vi "WVDIAL_2_OphirPM_v2.2_temp_tune.vi"() -> ()   [LabVIEW 2012]
uses:
  <vilib>/DAQmx/write.llb/DAQmx Write (Digital 1D Bool NChan 1Samp 1Line).vi
  <vilib>/DAQmx/miscellaneous.llb/DAQmx Fill In Error Info.vi
  under_development/AMCS_Data.vi
  <vilib>/Analysis/baseanly.llb/Mean (DBL).vi
  H2O_DIAL/LabVIEW-2012/Scalar_Data.vi
  H2O_DIAL/LabVIEW-2012/Bristol WM V2_31b/CLDevIFace.dll
  <vilib>/Analysis/NI_AALBase.lvlib
panel:
  out "AMCS_Profile":i32=256
  out "FileHour":i32=14
  out "L_Count":i32=93
  out "sigma_off_total":dbl[](array[numeric])=[5.314422064744898e-25, 5.279415210171283e-25, 5.244590126473598e-25, 5.20994645782043e-25, 5.175483839803292e-25, 5.1412018994858e-25, 5.1071002554464015e-25, 5.073178517853386e-25, 5.03943628848111e-25, 5.00587316081542e-25, 4.972488720065558e-25, 4.939282543255047e-25, 4.906254199251138e-25, 4.873403248837318e-25, 4.840729244783645e-25, 4.808231731862337e-25, 4.775910246962909e-25, 4.743764319119939e-25, 4.711793469569763e-25, 4.67999721182007e-25, 4.648375051724865e-25, 4.616926487509067e-25, 4.585651009873473e-25, 4.5545481020267065e-25, 4.52361723976039e-25, 4.49285789150236e-25, 4.4622695183981935e-25, 4.4318515743427665e-25, 4.40160350608453e-25, 4.371524753261039e-25, 4.3416147484733715e-25, 4.311872917347073e-25, 4.282298678608985e-25, 4.252891444145085e-25, 4.223650619059866e-25, 4.194575601773045e-25, 4.1656657840359355e-25, 4.136920551058964e-25, 4.1083392815469774e-25, 4.0799213477702186e-25, 4.05166611564624e-25, 4.0235729448119603e-25, 3.9956411886755236e-25, 3.967870194537133e-25, 3.9402593036058175e-25, 3.9128078511145925e-25, 3.885515166392363e-25, 3.858380572923638e-25, 3.8314033884573097e-25, 3.804582925057902e-25, 3.777918489222167e-25, 3.7514093819211588e-25, 3.7250548987302515e-25, 3.698854329879953e-25, 3.6728069603748863e-25, 3.646912070062639e-25, 3.62116893374067e-25, 3.595576821249159e-25, 3.5701349975624987e-25, 3.54484272290085e-25, 3.519699252824005e-25, 3.4947038383229287e-25, 3.469855725968371e-25, 3.445154157974239e-25, 3.420598372340985e-25, 3.3961876029492998e-25, 3.3719210796961754e-25, 3.347798028606905e-25, 3.323817671960307e-25, 3.2999792284274424e-25, 3.276281913173581e-25, 3.2527249380236306e-25, 3.2293075115830613e-25, 3.2060288393816585e-25, 3.1828881240106345e-25, 3.1598845652910105e-25, 3.1370173603985285e-25, 3.1142857040280253e-25, 3.091688788564397e-25, 3.069225804235743e-25, 3.0468959392679594e-25, 3.0246983800716816e-25, 3.002632311398086e-25, 2.980696916543016e-25, 2.958891377497247e-25, 2.9372148751466003e-25, 2.9156665894504283e-25, 2.89424569964799e-25, 2.8729513844353943e-25, 2.8517828221847843e-25, 2.8307391911095345e-25, 2.8098196695181605e-25, 2.7890234359787145e-25, 2.768349669545398e-25, 2.7477975499672548e-25, 2.727366257913024e-25, 2.7070549751927695e-25, 2.6868628849298454e-25, 2.6667891718580697e-25, 2.6468330224752645e-25, 2.6269936253020695e-25, 2.6072701711097747e-25, 2.587661853105292e-25, 2.5681678672237707e-25, 2.5487874122831935e-25, 2.529519690252841e-25, 2.5103639064422395e-25, 2.491319269774056e-25, 2.4723849929592074e-25, 2.453560292702316e-25, 2.434844389973349e-25, 2.416236510156665e-25, 2.3977358833193057e-25, 2.379341744342703e-25, 2.3610533331668965e-25, 2.3428698949963e-25, 2.3247906804276327e-25, 2.3068149456696086e-25, 2.288941952726386e-25, 2.2711709695222057e-25, 2.2535012700704786e-25, 2.235932134638202e-25, 2.21846284987704e-25, 2.201092708924474e-25, 2.183821011536941e-25, 2.1666470642157234e-25, 2.1495701802684266e-25, 2.1325896798994203e-25, 2.1157048902866705e-25, 2.098915145620556e-25, 2.082219787182239e-25, 2.0656181633016752e-25, 2.0491096294692994e-25, 2.0326935482406903e-25, 2.016369289258156e-25, 2.000136229269397e-25, 1.9839937520011981e-25, 1.9679412481191304e-25, 1.9519781152122327e-25, 1.9361037576226607e-25, 1.9203175863925343e-25, 1.9046190191099535e-25, 1.889007479817365e-25, 1.8734823987870487e-25, 1.8580432124512337e-25, 1.8426893631518894e-25, 1.8274202989506262e-25, 1.8122354735223218e-25, 1.7971343458200367e-25, 1.7821163799049579e-25, 1.767181044716152e-25, 1.752327813814955e-25, 1.737556165177881e-25, 1.7228655808367516e-25, 1.7082555467277782e-25, 1.693725552343894e-25, 1.6792750905240115e-25, 1.6649036571579248e-25, 1.650610750886898e-25, 1.6363958728621502e-25, 1.622258526492432e-25, 1.6081982171721664e-25, 1.594214451997735e-25, 1.580306739598529e-25, 1.5664745897902764e-25, 1.5527175135035033e-25, 1.5390350223941979e-25, 1.5254266288135843e-25, 1.5118918456024445e-25, 1.4984301858342265e-25, 1.4850411628570882e-25, 1.4717242900420903e-25, 1.4584790807687737e-25, 1.4453050483797776e-25, 1.4322017062029086e-25, 1.4191685674596558e-25, 1.4062051453739477e-25, 1.3933109532543182e-25, 1.3804855046380026e-25, 1.367728313352582e-25, 1.35503889384992e-25, 1.3424167612815224e-25, 1.3298614318833922e-25, 1.3173724233032037e-25, 1.3049492548807338e-25, 1.2925914480776576e-25, 1.2802985269669848e-25, 1.268070018646981e-25, 1.2559054538186517e-25, 1.2438043673528122e-25, 1.231766298852889e-25, 1.2197907933722819e-25, 1.207877402055392e-25, 1.1960256828031697e-25, 1.1842352011821407e-25, 1.172505531033491e-25, 1.160836255409088e-25, 1.149226967367832e-25, 1.1376772708317697e-25, 1.1261867814713535e-25, 1.1147551275979209e-25, 1.1033819510978471e-25, 1.0920669083258334e-25, 1.0808096709575008e-25, 1.069609927077414e-25, 1.0584673818555839e-25, 1.0473817586142326e-25, 1.0363527996489042e-25, 1.0253802670476093e-25, 1.0144639436397076e-25, 1.0036036335541817e-25, 9.927991632011449e-26, 9.820503819270136e-26, 9.713571625261393e-26, 9.607194020823438e-26, 9.501370223040411e-26, 9.396099700993619e-26, 9.291382180414976e-26, 9.187217645653203e-26, 9.083606343720884e-26, 8.980548784653646e-26, 8.878045744250468e-26, 8.776098262714437e-26, 8.674707644122939e-26, 8.573875455102998e-26, 8.473603522131269e-26, 8.373893928088327e-26, 8.274749007134821e-26, 8.17617134051572e-26, 8.078163749082583e-26, 7.980729286044041e-26, 7.883871229773624e-26, 7.78759307512813e-26, 7.691898521304032e-26, 7.596791464219395e-26, 7.502275983080843e-26, 7.408356329263953e-26, 7.315036913619158e-26, 7.222322292848408e-26, 7.130217155120976e-26, 7.038726307749827e-26, 6.947854659579743e-26, 6.857607208469795e-26, 6.767989024717408e-26, 6.679005234677889e-26, 6.59066100689568e-26, 6.502961534631894e-26, 6.415912020823876e-26, 6.329517661488074e-26, 6.243783631897422e-26, 6.158715068187244e-26, 6.074317054761003e-26, 5.99059460805025e-26, 5.907552662478026e-26, 5.825196055341633e-26, 5.743529514672476e-26, 5.662557645089932e-26, 5.582284915282987e-26, 5.502715646791743e-26, 5.423854001499785e-26, 5.345703972449223e-26, 5.268269372490484e-26, 5.191553826272697e-26, 5.1155607608625183e-26, 5.040293398726036e-26, 4.965754750357786e-26, 4.891947608760883e-26, 4.818874542569047e-26, 4.7465378935362823e-26, 4.674939770825742e-26, 4.604082049111456e-26, 4.533966365256215e-26, 4.464594117661327e-26, 4.395966464565719e-26, 4.328084324397715e-26, 4.260948375846483e-26, 4.1945590589570554e-26]
  out "sigma_on_total":dbl[](array[numeric])=[1.3869479575219666e-23, 1.3807437011066577e-23, 1.37449636602892e-23, 1.3682071082128486e-23, 1.3618770829571316e-23, 1.3555074444096617e-23, 1.3490993450978266e-23, 1.3426539354204636e-23, 1.3361723632425733e-23, 1.3296557734520282e-23, 1.3231053075022487e-23, 1.3165221030343146e-23, 1.3099072933460705e-23, 1.303262007172832e-23, 1.2965873680839169e-23, 1.2898844942369238e-23, 1.2831544980028457e-23, 1.2763984855328133e-23, 1.269617556404732e-23, 1.2628128033261598e-23, 1.2559853118242374e-23, 1.2491361598101514e-23, 1.2422664174044883e-23, 1.23537714654586e-23, 1.2284694007241841e-23, 1.221544224679423e-23, 1.2146026542230557e-23, 1.2076457158241087e-23, 1.2006744265409983e-23, 1.1936897936295945e-23, 1.1866928144067788e-23, 1.1796844760131547e-23, 1.1726657551867315e-23, 1.1656376181342888e-23, 1.1586010202384198e-23, 1.1515569060143322e-23, 1.1445062087730294e-23, 1.137449850683545e-23, 1.1303887424350273e-23, 1.1233237832313931e-23, 1.1162558605600282e-23, 1.1091858502038009e-23, 1.1021146159869723e-23, 1.0950430098256995e-23, 1.0879718715139568e-23, 1.0809020287073718e-23, 1.0738342968727736e-23, 1.0667694791434451e-23, 1.0597083663475774e-23, 1.0526517369210098e-23, 1.0456003568894101e-23, 1.0385549797974356e-23, 1.0315163467461895e-23, 1.024485186317274e-23, 1.0174622145845567e-23, 1.0104481351323143e-23, 1.003443639040392e-23, 9.964494049153228e-24, 9.89466098849997e-24, 9.824943745255963e-24, 9.755348732024939e-24, 9.685882237371367e-24, 9.616550426617036e-24, 9.547359341927676e-24, 9.47831490321052e-24, 9.40942290830694e-24, 9.340689033982913e-24, 9.272118836219597e-24, 9.203717751107802e-24, 9.135491095777061e-24, 9.067444068641131e-24, 8.999581750772038e-24, 8.931909106582237e-24, 8.864430984196331e-24, 8.797152117625856e-24, 8.730077126495636e-24, 8.663210517401465e-24, 8.596556685453482e-24, 8.530119914634811e-24, 8.46390437922709e-24, 8.397914144742156e-24, 8.332153169383828e-24, 8.266625304687613e-24, 8.201334296859706e-24, 8.136283788452192e-24, 8.071477318738257e-24, 8.006918325585158e-24, 7.942610146035729e-24, 7.878556018198735e-24, 7.81475908249396e-24, 7.751222382124728e-24, 7.687948864992263e-24, 7.624941385280568e-24, 7.562202703660279e-24, 7.499735489821076e-24, 7.43754232269632e-24, 7.375625692531723e-24, 7.31398800203366e-24, 7.25263156693754e-24, 7.191558618654768e-24, 7.130771304396952e-24, 7.070271689077592e-24, 7.010061756330106e-24, 6.950143409961645e-24, 6.890518475536768e-24, 6.831188701248949e-24, 6.772155758945719e-24, 6.713421246257091e-24, 6.654986687320795e-24, 6.596853534201044e-24, 6.539023168026952e-24, 6.481496900395139e-24, 6.424275974626182e-24, 6.3673615670133464e-24, 6.310754787803715e-24, 6.254456682823536e-24, 6.198468234566776e-24, 6.142790363279649e-24, 6.087423928166582e-24, 6.032369728708771e-24, 5.977628505719948e-24, 5.923200942640215e-24, 5.869087666691756e-24, 5.815289249902529e-24, 5.761806210124825e-24, 5.708639012516363e-24, 5.655788070409e-24, 5.603253746407087e-24, 5.551036353473567e-24, 5.4991361562284445e-24, 5.447553371437421e-24, 5.396288169850396e-24, 5.345340676553168e-24, 5.2947109721049526e-24, 5.244399093980751e-24, 5.1944050370119895e-24, 5.1447287546918326e-24, 5.09537016002838e-24, 5.0463291264942426e-24, 4.9976054888585635e-24, 4.949199044317764e-24, 4.901109553397718e-24, 4.853336740542285e-24, 4.805880295200359e-24, 4.758739872789894e-24, 4.711915095350015e-24, 4.6654055524798795e-24, 4.619210802353354e-24, 4.5733303718584396e-24, 4.527763758259087e-24, 4.482510429403448e-24, 4.437569824594334e-24, 4.392941355621808e-24, 4.3486244071369034e-24, 4.304618337478862e-24, 4.260922479571828e-24, 4.217536141448475e-24, 4.174458607031095e-24, 4.13168913672264e-24, 4.0892269680759445e-24, 4.0470713165327956e-24, 4.0052213761463945e-24, 3.96367631979338e-24, 3.9224353003739355e-24, 3.8814974509190375e-24, 3.840861885432312e-24, 3.800527699468413e-24, 3.760493970621977e-24, 3.72075975901009e-24, 3.681324108052961e-24, 3.642186044776093e-24, 3.603344580489083e-24, 3.564798711222146e-24, 3.526547418229872e-24, 3.4885896684839234e-24, 3.4509244152268236e-24, 3.413550598298677e-24, 3.376467144672314e-24, 3.339672968905001e-24, 3.3031669737165538e-24, 3.2669480501429536e-24, 3.231015078099695e-24, 3.1953669267941692e-24, 3.1600024551943975e-24, 3.1249205122895757e-24, 3.0901199376068864e-24, 3.055599561330377e-24, 3.0213582050544584e-24, 2.987394681822326e-24, 2.953707796666617e-24, 2.92029634676618e-24, 2.8871591220256764e-24, 2.854294905098644e-24, 2.821702472007482e-24, 2.7893805922154235e-24, 2.7573280291639967e-24, 2.725543540222118e-24, 2.694025877377622e-24, 2.662773787176486e-24, 2.6317860112783244e-24, 2.60106128650067e-24, 2.5705983450847046e-24, 2.5403959152174938e-24, 2.5104527209047027e-24, 2.4807674825825997e-24, 2.4513389169868365e-24, 2.4221657375927964e-24, 2.3932466549360318e-24, 2.3645803764788273e-24, 2.3361656072702794e-24, 2.308001049756091e-24, 2.2800854041775233e-24, 2.2524173687645203e-24, 2.2249956398311676e-24, 2.197818912100556e-24, 2.170885878654516e-24, 2.1441952314281124e-24, 2.1177456610619372e-24, 2.091535857292432e-24, 2.065564508979104e-24, 2.0398303043057066e-24, 2.014331931015518e-24, 1.9890680763476753e-24, 1.9640374273914704e-24, 1.9392386711399865e-24, 1.9146704945060966e-24, 1.890331584774096e-24, 1.8662206293279557e-24, 1.8423363160920896e-24, 1.8186773334553743e-24, 1.795242370503451e-24, 1.7720301170920184e-24, 1.749039263883513e-24, 1.7262685025646166e-24, 1.703716525946266e-24, 1.6813820279212657e-24, 1.6592637036703435e-24, 1.6373602498566653e-24, 1.6156703644751474e-24, 1.5941927471134708e-24, 1.572926098969147e-24, 1.5518691229974072e-24, 1.5310205238931107e-24, 1.510379008202476e-24, 1.48994328452232e-24, 1.4697120633218853e-24, 1.44968405723214e-24, 1.4298579810194845e-24, 1.410232551681262e-24, 1.3908064884217362e-24, 1.371578512888116e-24, 1.3525473490547908e-24, 1.333711723340262e-24, 1.315070364690135e-24, 1.2966220046291443e-24, 1.2783653772848224e-24, 1.2602992193856838e-24, 1.2424222704417105e-24, 1.2247332727096541e-24, 1.207230971188227e-24, 1.1899141137880397e-24, 1.1727814512227674e-24, 1.1558317371980456e-24, 1.1390637283275014e-24, 1.1224761842431351e-24, 1.1060678675840506e-24, 1.0898375441228311e-24, 1.0737839826609285e-24, 1.057905955131391e-24, 1.0422022366512468e-24, 1.0266716055496742e-24, 1.0113128433115541e-24, 9.96124734733142e-25, 9.811060678425485e-25, 9.662556339483166e-25, 9.515722277242587e-25, 9.370546471719464e-25]
  out "background start":u32=254
  in  "Tab Control 2":enum32{"WV ND Narrow", "WV ND Wide"}(tab)
  out "Water Vapor Number Density":dbl[][](graph)=[[2.6979991604572735, 2.9593143915657074, 2.797449584571317, 2.404658952819358, 2.3195212072555154, 2.5116972565306184, 2.4617308913751637, 2.4391959235044225, 2.6692800938976244, 2.741253898038124, 2.644730576020495, 2.3610708500867044, 2.1476349969634225, 2.2002457128655424, 2.4968510217618705, 2.554578876255192, 2.0454846988586315, 1.8023042055354455, 1.9720735301407404, 1.8926202748500127, 1.7837401064253728, 2.0676382839883733, 2.08031025810689, 1.773643007504944, 1.6546102834122778, 1.6279557460647043, 1.6011324659921025, 1.0021875680291408, 0.41374082119247085, 0.4527192082231668, 2.3516701899198997, 4.374135424821069, 0.39214939184879105, -5.085477705081822, -0.6454633347922013, 8.345959457204707, 1.182839582693342, -1.7003003047291725, 6.536266318699054, -2.327645608957367, 2.797319081322348, 0.10721086091200081, 0.8678650894368296, -0.292961171425824, -1.2405862868143065, 0.08002385618879078, 1.1423277801066902, 0.8810874015440164, 1.166620200538605, 1.1437670100476367, 3.3905729378505236, 5.02328449196602, 2.4176112321239813, 1.7373231866673655, 0.21866881048224668, -0.6606779691744664, 0.8866008233295397, 5.183030048638962, 7.624360936578197, -2.561027107157697, -4.6351658542352805, -4.1844318407939305, -2.990804811815481, -0.08651792227088426, 2.1460065959464, 5.64031573417192, 7.404702135500966, 1.3666150911852348, -7.13957308573761, 0.3596983598284657, -3.2319741125605272, -5.382731401201804, -3.658947755685539, -6.466561447894286, -2.5894001538271456, -3.5936030711328533, -9.45888310637412, 5.337453776109291, 2.523301465289049, -0.4444154792139517, 3.9416736698791515, -0.31355796660419666, -1.8373168582667905, 0.9955190223681669, -1.089077347483283, -6.281856233414937, 6.257260372926666, -13.655858715766612, 5.830204522057969, 9.609389261892614, -3.924288936198821, 4.924456138151559, 4.670517947496226, 7.722670563052783, 12.254047544716892, 9.745839454508765, -3.8105997194228154, 0.4890661768678136, 11.894606542817344, -16.259140432303216, 12.884851240924808, -9.074814833037872, -0.07410598267861004, 13.032695980210102, -15.347711948234926, -2.2813575808650772, -0.37180440848685486, 19.946704578086855, -16.686062841021247, -9.894667631120459, -20.995606668812822, -2.2526592621705586, -16.3908377368364, -21.31038895828113, 32.72210513307602, -9.717538636026543, -9.890235552804324, -26.917838345809066, -11.15341741047493, 16.822178540332708, 11.164934912668619, 8.976059522967718, 16.44419788472998, 5.521276634043085, -27.348050690597656, 3.2607914106748015, 10.64540411389454, 26.35964743727274, 8.217737459322414, -2.1446882284347537, -1.6240017477306874, 0.8694361012620837, 0.2753212901219622, -2.017177128570476, -1.7367818265406356, 2.738866245516143, -2.2576465932228675, -18.144499153577325, -3.4713944166922777, 0.025358387211094534, 3.8925246272702494, 2.6620676732061166, -5.242800367205337, -4.258745982226573, -0.746059052925772, -0.05154706973106406, 2.990291161294011, 8.0729458717512, 8.116266129237458, 6.226968559806926, -17.485848033155328, -7.175474933960434, 9.897116918290264, -5.562391740806701, -28.26312520479269, -37.18466121475089, 3.0379212507936595, -49.25326375258036, -49.55319390746631, -75.79505294806995, -31.800298571915437, -21.323573928947045, 6.170114127015452, -32.59512054829957, 41.14643545755569, 72.32002090526684, -19.19621968895502, 76.64601181450533, 40.58764334357079, 43.20212176036005, 30.51415344385976, -18.900153250831522, -12.69555435106068, 40.90487604463205, -43.90464231635574, -71.87217734267412, -85.25284930724254, -98.86218389373931, -37.211623515974594, -4.660221249767364, -8.30223960482317, -78.11880710674619, -52.936142176356334, 10.739065034224021, 27.17659341050922, 43.27549838133942, 78.6390303110269, 31.63798764245529, 22.840921363665966, -15.424992732340193, -67.11504703685894, 95.28139075009446, 47.665759432899335, 39.75623750944128, 12.07897488147926, -13.595402683839163, -16.244355600957185, 39.56289276585016, -58.46898177728697, -5.705909600699701, 36.35847497013099, -103.67852139769494, -65.209907256163, -117.84105778782569, -37.196968834476365, -4.511454495944519, 38.957598425261125, -28.163785822065798, 55.90715401535311, 20.281060958402115, 100.0959062964011, 29.293400539831783, 55.15876114229656, -65.2961513762635, -4.429021621104553, -22.382554280854816, 15.842494942030372, -29.55499174522829, 7.668766094225895, 50.010508877808284, -88.02683061785386, 30.08347486970615, 106.39829367365633, 145.2321906759042, -1.858002730325935, -18.46040484465744, 1.3292343668491104, 29.845298073762176, 20.54006800357979, 6.775417401267568, 108.55704162770199, 21.35361701301774, -22.183740735151503, 26.424235225087745, -0.2082268013256196, 11.16104876593104, 74.9397615826961, 0.2512828787561202, -18.73257114374409, -9.174859609068479, -0.6049319170897494, 41.81659884060494, -105.33239517840579, -50.40203588046909, 294.29886187228936, 68.70660941139782, -104.26441281434118, -17.894724880282443, -14.734992121972157, -79.59667884368375, -149.05753799401518, 30.40850937412097, -4.110243462106567, -30.737568940274127, -355.33349697162674, -84.80653337159367, 60.380833898611876, -72.78540457827825, -55.41791512520111, -117.56784011631594, 73.39110087767413, 236.13722109125632, -50.17444896136822, 72.78920342275046, -77.32879365741358, -50.85238879922648, -149.21416360461436, 57.54491199600477, 205.8524361343854, 232.8390700997829, -110.53199462104917, -378.03756929059244, -27.712093052120554, -149.1541222983105, 54.68721852689611, -11.376835333855148, 0.0, 0.0, 0.0, 0.0]]
  out "Water Vapor Number Density 2":dbl[][](graph)=[[nan, nan, nan, nan, nan, nan, nan, nan, nan, nan, nan, nan, nan, nan, nan, nan, nan, nan, nan, nan, nan, nan, nan, nan, nan, nan, nan, nan, nan, nan, nan, nan, nan, nan, nan, nan, nan, nan, nan, nan, nan, nan, nan, nan, nan, nan, nan, nan, nan, nan, nan, nan, nan, nan, nan, nan, nan, nan, nan, nan, nan, nan, nan, nan, nan, nan, nan, nan, nan, nan, nan, nan, nan, nan, nan, nan, nan, nan, nan, nan, nan, nan, nan, nan, nan, nan, nan, nan, nan, nan, nan, nan, nan, nan, nan, nan, nan, nan, nan, nan, nan, nan, nan, nan, nan, nan, nan, nan, nan, nan, nan, nan, nan, nan, nan, nan, nan, nan, nan, nan, nan, nan, nan, nan, nan, nan, nan, nan, nan, nan, nan, nan, nan, nan, nan, nan, nan, nan, nan, nan, nan, nan, nan, nan, nan, nan, nan, nan, nan, nan, nan, nan, nan, nan, nan, nan, nan, nan, nan, nan, nan, nan, nan, nan, nan, nan, nan, nan, nan, nan, nan, nan, nan, nan, nan, nan, nan, nan, nan, nan, nan, nan, nan, nan, nan, nan, nan, nan, nan, nan, nan, nan, nan, nan, nan, nan, nan, nan, nan, nan, nan, nan, nan, nan, nan, nan, nan, nan, nan, nan, nan, nan, nan, nan, nan, nan, nan, nan, nan, nan, nan, nan, nan, nan, nan, nan, nan, nan, nan, nan, nan, nan, nan, nan, nan, nan, nan, nan, nan, nan, nan, nan, nan, nan, nan, nan, nan, nan, nan, nan, nan, nan, nan, nan, nan, nan, nan, nan, nan, nan, nan, nan, nan, nan, nan, nan, nan, nan, nan, nan, nan, nan, nan, nan, nan, nan, 0.0, 0.0, 0.0, 0.0]] caption="Water Vapor Number Density"
  out "RingBuffer offline near":dbl[][](array[numeric])
  out "RingBuffer aerosol near":dbl[][](array[numeric])
  in  "LOWER DISPLAY TAB":T1(tab)=enum."Raw Counts Narrow"
  out "NRB":dbl[][](graph)=[[0.00046653927091916777, 0.0026614448003019955, 0.00799000665119036, 0.017338442995885873, 0.030659739318508464, 0.048690127127963834, 0.07257190803169539, 0.1022875233425713, 0.13895426462578678, 0.18353308368702612, 0.2374733807532343, 0.29827916455644055, 0.36303037111961745, 0.4387277399880996, 0.5296240484959289, 0.6448056167411246, 0.7968692742688123, 0.986211936517738, 1.2272580015909782, 1.5045937819461137, 1.6804030717427192, 1.6930670107515053, 1.7186662137889164, 1.8220745936144405, 1.921986223781103, 2.0763561968674273, 2.2958981573467914, 2.3486417326554654, 2.047301484620606, 1.411776366563831, 0.7124512356303606, 0.3105075790623782, 0.2141663700100353, 0.2121969246397393, 0.19959202927447903, 0.1761001939839144, 0.16578999175180362, 0.17348619277005686, 0.17737239738890392, 0.19260470674885563, 0.18387703555551488, 0.1683847338008346, 0.18113483921557574, 0.19140229669855557, 0.20519979528052695, 0.23908830659210373, 0.24929346127216373, 0.21410890747194383, 0.19758618909133507, 0.19339446633371923, 0.1918349029632283, 0.1666024208595111, 0.17274180772746983, 0.18857177921404147, 0.16091218794964157, 0.15551975294417666, 0.19172069794668137, 0.21550100504467, 0.1939605427805015, 0.15555508504784912, 0.15837969068596502, 0.17392434388819766, 0.17375269565396587, 0.18099628966643178, 0.1552686332629994, 0.1871983829024575, 0.19326554001157917, 0.1759961805666762, 0.20702641454615772, 0.17230592991361512, 0.15624762843920986, 0.1362276160575669, 0.11219171781224463, 0.16126344429341657, 0.17622056993508411, 0.13652363159974298, 0.13828342852020437, 0.13106340939532152, 0.13053713937048633, 0.1098155705898619, 0.12618801482529873, 0.16498428580884197, 0.16768457837801556, 0.1613926144792111, 0.1467353339521328, 0.14687923449528653, 0.09921420381956712, 0.028623899549958025, 0.09638828573179213, 0.13898533152779396, 0.0993106431198225, 0.1341337314641019, 0.08578445870698116, 0.14988499019441937, 0.24740804086795487, 0.23532835084484116, 0.1365893927881256, 0.09149807112681532, 0.16145936216816204, 0.17178252103390232, 0.15986434455570978, 0.10909509408905861, 0.11830283727003509, 0.09754229119527288, 0.0629700043568801, 0.16201238738941418, 0.1861436261348872, 0.21566036035440786, 0.19200480679779117, 0.1462942034668786, 0.19646330323797864, 0.17424490794472436, 0.24358767939255435, 0.15560140404548056, -0.03262194064558316, -0.05030318579422492, 0.063722224941549, -0.0016563122467756772, -0.02246353446437762, 0.10337828990755542, 0.1116973847636031, 0.1441309624918215, 0.12962967679387316, 0.13565725674439336, 0.04155142740366882, 0.3597156443785714, 0.9053359221232993, 1.3274351658049444, 1.5516506598520667, 1.6890247548740251, 1.456939178163056, 0.8251997771899959, 0.5264651467937713, 0.5474151217059147, 1.153592838836607, 2.7245958688554976, 5.9590100032700875, 10.358807868304037, 13.752597951922784, 13.321173266620074, 9.929368166634307, 8.319699656050076, 10.215466411241565, 11.264037378065957, 8.239090023036898, 3.8676449804333157, 1.8091720120289554, 1.5417339483555401, 1.184874433985245, 1.1964269980813527, 1.8071508438115211, 2.8350889457012673, 3.31983490827713, 2.551437870592605, 1.1740390978029294, 0.4566254679466681, 0.14705412703589116, 0.1748216055487878, 0.19336548065559225, -0.10070999224246821, -0.00916904547514361, 0.05489969276362185, -0.0613790147296684, -0.008461508611298307, 0.10489231744081019, 0.2253241019004552, 0.2744321054481327, 0.1556808399563599, 0.14133368334941515, 0.10060220872991148, 0.09835652831180781, 0.31658200601100306, 0.47195886105167817, 0.4276641830684275, 0.15394419938215426, -0.03701654742796507, 0.0630851327862899, -0.039102373767677445, 0.10652094665295668, 0.10264304191186455, 0.18839860179433146, 0.2377987829790185, -0.1337107048088187, 0.009220418178048348, 0.041462246018112034, -0.10564267279908282, 0.12514963530437614, 0.013774666881661655, -0.30544644422181294, -0.08551608415499386, 0.10272375530400045, 0.19251893526497038, 0.319889127727876, -0.06632874219283735, -0.3987896018285478, -0.017346889667260754, 0.41454046411268386, 0.4287323252398325, 0.27654890615479055, 0.0069807213602538455, 0.052106026597721615, 0.07897094487093263, -0.0694008008611362, -0.17674330597107643, -0.14394925906419756, 0.13443704094357667, 0.31851437756105405, -0.03985065387486617, -0.3248039530724683, 0.008559054170191926, 0.08529365932724306, 0.09225944268644928, -0.016936024365819886, 0.2839683030158373, 0.44400723102129164, 0.1797559582192265, 0.24776078000505974, -0.14047093671496036, -0.4898589719637731, -0.03321834143453104, 0.2225764985272629, 0.12141788420013612, 0.23732622403377998, 0.3091639446236378, 0.37037323028296343, 0.13182866468330257, -0.08073210235332377, -0.0895812330679099, -0.08729083537973405, 0.17172702391260303, 0.06151272265106227, 0.11785957903150333, 0.27183497399482814, 0.5377361440387042, 0.2894881510858271, 0.009719956422017425, 0.23179347279449192, -0.18959136484778202, -0.27164793180882657, 0.11035050374540555, 0.03627218441554687, -0.5729506651960073, -0.7197745629796234, -0.5020978864046269, -0.26197225331804413, -0.2842416644426923, -0.12303750456090687, -0.03860209607355206, -0.20873459471373904, 0.106286853878823, 0.056601357578755326, -0.20634031751796159, 0.3367860809816278, 0.360913317766556, 0.052058689588379094, -0.05139020644874281, -0.19781130293363244, -0.14856534214258266, 0.005144708507677107, 0.20622067097216687, 0.1691582294324484, 0.33565453726380606, 0.30032763979924, -0.4228041465415953, -0.586748613218039, 0.10509902204196496, -0.15353229797165785, -0.7209430470045907, -0.1827390073296543, 0.11113626218212269, -0.24868566608054246, 0.13450151047086945, 0.4665084611774521, 0.30834835440009084, -0.14067735872021378, -0.35630589536410423, 0.046416854918681326, 0.0, 0.0, 0.0]] caption="Water Vapor Number Density"
  out "NRB 2":dbl[][](graph) caption="Water Vapor Number Density"
  out "raw counts":dbl[][](graph)=[[342.03999999999996, 498.03999999999996, 667.04, 800.04, 1022.04, 1083.04, 1284.04, 1434.04, 1514.04, 1579.04, 1641.04, 1669.04, 1825.04, 1971.04, 1925.04, 2051.04, 2144.04, 2361.04, 2590.04, 2967.04, 3312.04, 3169.04, 2904.04, 2546.04, 2575.04, 2469.04, 2578.04, 3175.04, 3166.04, 2114.04, 1163.04, 339.03999999999996, 161.03999999999996, 176.03999999999996, 92.03999999999996, 188.03999999999996, 84.03999999999996, 121.03999999999996, 103.03999999999996, 90.03999999999996, 156.03999999999996, 130.03999999999996, 93.03999999999996, 116.03999999999996, 139.03999999999996, 126.03999999999996, 154.03999999999996, 91.03999999999996, 109.03999999999996, 58.039999999999964, 54.039999999999964, 77.03999999999996, 5.039999999999964, 14.039999999999964, 158.03999999999996, -64.96000000000004, 44.039999999999964, 54.039999999999964, 26.039999999999964, 26.039999999999964, 52.039999999999964, 66.03999999999996, 71.03999999999996, 24.039999999999964, 79.03999999999996, 77.03999999999996, 45.039999999999964, 7.039999999999964, -19.960000000000036, 24.039999999999964, 14.039999999999964, 40.039999999999964, 47.039999999999964, -10.960000000000036, -29.960000000000036, 79.03999999999996, 4.039999999999964, 96.03999999999996, 23.039999999999964, -35.960000000000036, 42.039999999999964, -28.960000000000036, 49.039999999999964, 20.039999999999964, -15.960000000000036, -16.960000000000036, 3.0399999999999636, 57.039999999999964, -6.960000000000036, 16.039999999999964, 34.039999999999964, -5.960000000000036, 24.039999999999964, 27.039999999999964, 12.039999999999964, -78.96000000000004, -29.960000000000036, -1.9600000000000364, 0.03999999999996362, 15.039999999999964, 76.03999999999996, -37.960000000000036, 35.039999999999964, 6.039999999999964, -0.9600000000000364, -71.96000000000004, 12.039999999999964, 82.03999999999996, 57.039999999999964, 43.039999999999964, 14.039999999999964, -42.960000000000036, 4.039999999999964, -26.960000000000036, 28.039999999999964, -35.960000000000036, -31.960000000000036, 13.039999999999964, -67.96000000000004, -73.96000000000004, 15.039999999999964, -22.960000000000036, -21.960000000000036, 32.039999999999964, -80.96000000000004, 6.039999999999964, 35.039999999999964, 77.03999999999996, 17.039999999999964, 52.039999999999964, 63.039999999999964, 55.039999999999964, 52.039999999999964, 4.039999999999964, 12.039999999999964, 79.03999999999996, 122.03999999999996, 368.03999999999996, 606.04, 607.04, 506.03999999999996, 233.03999999999996, 293.03999999999996, 312.03999999999996, 364.03999999999996, 257.03999999999996, -12.960000000000036, 13.039999999999964, 22.039999999999964, 48.039999999999964, 146.03999999999996, 137.03999999999996, 125.03999999999996, 115.03999999999996, 36.039999999999964, -39.960000000000036, -9.960000000000036, -19.960000000000036, 19.039999999999964, -11.960000000000036, 28.039999999999964, -43.960000000000036, 3.0399999999999636, -24.960000000000036, 16.039999999999964, -58.960000000000036, -5.960000000000036, 35.039999999999964, 44.039999999999964, -19.960000000000036, -40.960000000000036, -1.9600000000000364, 63.039999999999964, -33.960000000000036, 21.039999999999964, -23.960000000000036, -43.960000000000036, -54.960000000000036, -106.96000000000004, -19.960000000000036, -77.96000000000004, -32.960000000000036, -5.960000000000036, -10.960000000000036, 33.039999999999964, 10.039999999999964, -22.960000000000036, 46.039999999999964, 83.03999999999996, 58.039999999999964, 24.039999999999964, 13.039999999999964, 2.0399999999999636, 43.039999999999964, 15.039999999999964, -58.960000000000036, 62.039999999999964, 55.039999999999964, -53.960000000000036, 32.039999999999964, 9.039999999999964, -55.960000000000036, 5.039999999999964, -9.960000000000036, -5.960000000000036, 3.0399999999999636, -8.960000000000036, 21.039999999999964, 7.039999999999964, 57.039999999999964, 15.039999999999964, -3.9600000000000364, -6.960000000000036, -13.960000000000036, 4.039999999999964, 58.039999999999964, -9.960000000000036, 29.039999999999964, -16.960000000000036, -46.960000000000036, 51.039999999999964, 12.039999999999964, -62.960000000000036, -3.9600000000000364, -13.960000000000036, -10.960000000000036, 18.039999999999964, 47.039999999999964, -18.960000000000036, -34.960000000000036, -9.960000000000036, 8.039999999999964, -44.960000000000036, -20.960000000000036, 1.0399999999999636, -27.960000000000036, 36.039999999999964, 45.039999999999964, -24.960000000000036, -13.960000000000036, -16.960000000000036, -26.960000000000036, -20.960000000000036, -8.960000000000036, 25.039999999999964, -26.960000000000036, -4.960000000000036, 53.039999999999964, -41.960000000000036, 9.039999999999964, 14.039999999999964, -21.960000000000036, -55.960000000000036, -18.960000000000036, -3.9600000000000364, 32.039999999999964, -38.960000000000036, 24.039999999999964, 4.039999999999964, -16.960000000000036, -28.960000000000036, -34.960000000000036, 18.039999999999964, 30.039999999999964, 9.039999999999964, -49.960000000000036, 41.039999999999964, -50.960000000000036, -39.960000000000036, 23.039999999999964, 41.039999999999964, 37.039999999999964, 13.039999999999964, 5.039999999999964, 7.039999999999964, 23.039999999999964, 1.0399999999999636, -64.96000000000004, 21.039999999999964, 0.0]] caption="Water Vapor Number Density"
  out "raw counts near":dbl[][](graph) caption="Water Vapor Number Density"
  out "Aerosol Smoothed 2":dbl[](array[numeric])
  out "Off-Line Smoothed 2":dbl[](array[numeric])
  out "Off-Line Bin Readings 2":dbl[](array[numeric])
  out "On-Line Smoothed 2":dbl[](array[numeric])
  out "On-Line Bin Readings 2":dbl[](array[numeric])
  in  "stop":bool
  in  "Reset Average":bool=TRUE
  in  "Save Data?":bool=TRUE
  in  "Collect Data?":bool=TRUE
  in  "Tab Control":T2(tab)=enum."NRB"
  out "Water Vapor Number Density  2":cluster{"Y":dbl[], "Y":dbl[]}[](graph)=[{"Y"=array[276 elements], "Y"=array[280 elements]}, {"Y"=[nan, nan, nan, nan, nan, nan, nan, nan, nan, nan, nan, nan, nan, nan, nan, nan, nan, nan, nan, nan, nan, nan, nan, nan, nan, nan, nan, nan, nan, nan, nan, nan, nan, nan, nan, nan, nan, nan, nan, nan, nan, nan, nan, nan, nan, nan, nan, nan, nan, nan, nan, nan, nan, nan, nan, nan, nan, nan, nan, nan, nan, nan, nan, nan, nan, nan, nan, nan, nan, nan, nan, nan, nan, nan, nan, nan, nan, nan, nan, nan, nan, nan, nan, nan, nan, nan, nan, nan, nan, nan, nan, nan, nan, nan, nan, nan, nan, nan, nan, nan, nan, nan, nan, nan, nan, nan, nan, nan, nan, nan, nan, nan, nan, nan, nan, nan, nan, nan, nan, nan, nan, nan, nan, nan, nan, nan, nan, nan, nan, nan, nan, nan, nan, nan, nan, nan, nan, nan, nan, nan, nan, nan, nan, nan, nan, nan, nan, nan, nan, nan, nan, nan, nan, nan, nan, nan, nan, nan, nan, nan, nan, nan, nan, nan, nan, nan, nan, nan, nan, nan, nan, nan, nan, nan, nan, nan, nan, nan, nan, nan, nan, nan, nan, nan, nan, nan, nan, nan, nan, nan, nan, nan, nan, nan, nan, nan, nan, nan, nan, nan, nan, nan, nan, nan, nan, nan, nan, nan, nan, nan, nan, nan, nan, nan, nan, nan, nan, nan, nan, nan, nan, nan, nan, nan, nan, nan, nan, nan, nan, nan, nan, nan, nan, nan, nan, nan, nan, nan, nan, nan, nan, nan, nan, nan, nan, nan, nan, nan, nan, nan, nan, nan, nan, nan, nan, nan, nan, nan, nan, nan, nan, nan, nan, nan, nan, nan, nan, nan, nan, nan, nan, nan, nan, nan, nan, nan], "Y"=array[280 elements]}]
  out "Absolute Humidity":cluster{"Y":dbl[], "Y":dbl[]}[](graph)=[{"Y"=array[276 elements], "Y"=array[280 elements]}, {"Y"=[nan, nan, nan, nan, nan, nan, nan, nan, nan, nan, nan, nan, nan, nan, nan, nan, nan, nan, nan, nan, nan, nan, nan, nan, nan, nan, nan, nan, nan, nan, nan, nan, nan, nan, nan, nan, nan, nan, nan, nan, nan, nan, nan, nan, nan, nan, nan, nan, nan, nan, nan, nan, nan, nan, nan, nan, nan, nan, nan, nan, nan, nan, nan, nan, nan, nan, nan, nan, nan, nan, nan, nan, nan, nan, nan, nan, nan, nan, nan, nan, nan, nan, nan, nan, nan, nan, nan, nan, nan, nan, nan, nan, nan, nan, nan, nan, nan, nan, nan, nan, nan, nan, nan, nan, nan, nan, nan, nan, nan, nan, nan, nan, nan, nan, nan, nan, nan, nan, nan, nan, nan, nan, nan, nan, nan, nan, nan, nan, nan, nan, nan, nan, nan, nan, nan, nan, nan, nan, nan, nan, nan, nan, nan, nan, nan, nan, nan, nan, nan, nan, nan, nan, nan, nan, nan, nan, nan, nan, nan, nan, nan, nan, nan, nan, nan, nan, nan, nan, nan, nan, nan, nan, nan, nan, nan, nan, nan, nan, nan, nan, nan, nan, nan, nan, nan, nan, nan, nan, nan, nan, nan, nan, nan, nan, nan, nan, nan, nan, nan, nan, nan, nan, nan, nan, nan, nan, nan, nan, nan, nan, nan, nan, nan, nan, nan, nan, nan, nan, nan, nan, nan, nan, nan, nan, nan, nan, nan, nan, nan, nan, nan, nan, nan, nan, nan, nan, nan, nan, nan, nan, nan, nan, nan, nan, nan, nan, nan, nan, nan, nan, nan, nan, nan, nan, nan, nan, nan, nan, nan, nan, nan, nan, nan, nan, nan, nan, nan, nan, nan, nan, nan, nan, nan, nan, nan, nan], "Y"=array[280 elements]}]
  out "NRB plot":cluster{"Y":dbl[], "Y":dbl[]}[](graph)
  in  "background length":i32=25
  out "Correction":cluster{"Y":dbl[], "Y":dbl[]}[](graph)=[{"Y"=array[277 elements], "Y"=array[280 elements]}, {"Y"=[1.0, 1.0, 1.0, 1.0, 1.0, 1.0, 1.0, 1.0, 1.0, 1.0, 1.0, 1.0, 1.0, 1.0, 1.0, 1.0, 1.0, 1.0, 1.0, 1.0, 1.0, 1.0, 1.0, 1.0, 1.0, 1.0, 1.0, 1.0, 1.0, 1.0, 1.0, 1.0, 1.0, 1.0, 1.0, 1.0, 1.0, 1.0, 1.0, 1.0, 1.0, 1.0, 1.0, 1.0, 1.0, 1.0, 1.0, 1.0, 1.0, 1.0, 1.0, 1.0, 1.0, 1.0, 1.0, 1.0, 1.0, 1.0, 1.0, 1.0, 1.0, 1.0, 1.0, 1.0, 1.0, 1.0, 1.0, 1.0, 1.0, 1.0, 1.0, 1.0, 1.0, 1.0, 1.0, 1.0, 1.0, 1.0, 1.0, 1.0, 1.0, 1.0, 1.0, 1.0, 1.0, 1.0, 1.0, 1.0, 1.0, 1.0, 1.0, 1.0, 1.0, 1.0, 1.0, 1.0, 1.0, 1.0, 1.0, 1.0, 1.0, 1.0, 1.0, 1.0, 1.0, 1.0, 1.0, 1.0, 1.0, 1.0, 1.0, 1.0, 1.0, 1.0, 1.0, 1.0, 1.0, 1.0, 1.0, 1.0, 1.0, 1.0, 1.0, 1.0, 1.0, 1.0, 1.0, 1.0, 1.0, 1.0, 1.0, 1.0, 1.0, 1.0, 1.0, 1.0, 1.0, 1.0, 1.0, 1.0, 1.0, 1.0, 1.0, 1.0, 1.0, 1.0, 1.0, 1.0, 1.0, 1.0, 1.0, 1.0, 1.0, 1.0, 1.0, 1.0, 1.0, 1.0, 1.0, 1.0, 1.0, 1.0, 1.0, 1.0, 1.0, 1.0, 1.0, 1.0, 1.0, 1.0, 1.0, 1.0, 1.0, 1.0, 1.0, 1.0, 1.0, 1.0, 1.0, 1.0, 1.0, 1.0, 1.0, 1.0, 1.0, 1.0, 1.0, 1.0, 1.0, 1.0, 1.0, 1.0, 1.0, 1.0, 1.0, 1.0, 1.0, 1.0, 1.0, 1.0, 1.0, 1.0, 1.0, 1.0, 1.0, 1.0, 1.0, 1.0, 1.0, 1.0, 1.0, 1.0, 1.0, 1.0, 1.0, 1.0, 1.0, 1.0, 1.0, 1.0, 1.0, 1.0, 1.0, 1.0, 1.0, 1.0, 1.0, 1.0, 1.0, 1.0, 1.0, 1.0, 1.0, 1.0, 1.0, 1.0, 1.0, 1.0, 1.0, 1.0, 1.0, 1.0, 1.0, 1.0, 1.0, 1.0, 1.0, 1.0, 1.0, 1.0, 1.0, 1.0, 1.0, 1.0, 1.0, 1.0, 1.0, 1.0, 1.0, 1.0, 1.0, 1.0, 1.0, 1.0, 1.0, 1.0, 1.0, 1.0, 1.0, 1.0, 1.0, 1.0, 1.0, 1.0, 1.0, 1.0, 1.0], "Y"=array[280 elements]}]
  in  "dead time":dbl=3.7e-08
  out "Optical Depth":cluster{"Y":dbl[], "Y":dbl[]}[](graph) caption="XY Graph"
  out "RingBuffer offline far":dbl[][](array[numeric])
  out "RingBuffer aerosol far":dbl[][](array[numeric])
  in  "Weather":T3(tab)=enum."Pulse Energy (Micro Joule)"
  out "Temperature (C)":dbl(graph)=25.519230769230774
  out "Pressure (mb)":dbl(graph)=977.3351648351648
  out "Relative Humdity (%)":dbl(graph)=37.15201465201466
  out "Pulse Energy (Micro Joule)":cluster{dbl}(graph)={4.971428571428571}
  in  "PRF (kHz)":dbl=7.0
  in  "energy scale":dbl=0.05
  out "?":cluster{"mean":dbl, "mean":dbl}(graph)={"mean"=232392.0, "mean"=0.0}
  out "Index":i32=94
  out "Aerosol Smoothed":dbl[](array[numeric])=[409.8779310344828, 583.791724137931, 777.8089655172414, 948.2055172413793, 1072.1020689655172, 1181.3779310344828, 1292.5848275862072, 1393.7917241379314, 1494.8951724137935, 1598.0848275862072, 1707.4813793103453, 1800.8606896551728, 1866.6365517241384, 1943.964137931035, 2042.72275862069, 2183.481379310345, 2386.6020689655174, 2629.74, 2930.360689655172, 3234.7572413793105, 3275.8262068965514, 3013.3262068965514, 2803.1710344827584, 2730.843448275862, 2656.25724137931, 2653.171034482758, 2719.050344827586, 2588.9468965517244, 2111.464137931035, 1368.2400000000002, 650.1537931034482, 266.6882758620689, 173.08482758620687, 161.56758620689658, 143.4296551724138, 119.63655172413795, 106.63655172413795, 105.79172413793104, 102.68827586206896, 105.99862068965518, 96.32620689655172, 84.06758620689655, 86.27448275862069, 87.06758620689655, 89.24000000000001, 99.49862068965517, 99.37793103448276, 81.84344827586207, 72.48137931034483, 68.13655172413793, 64.96413793103449, 54.27448275862069, 54.17103448275862, 56.964137931034486, 46.860689655172415, 43.68827586206896, 51.98137931034483, 56.429655172413796, 49.0848275862069, 38.06758620689655, 37.49862068965517, 39.860689655172415, 38.56758620689655, 38.92965517241379, 32.377931034482756, 37.860689655172415, 37.929655172413796, 33.53310344827587, 38.308965517241376, 30.981379310344828, 27.308965517241383, 23.15379310344828, 18.55034482758621, 25.946896551724137, 27.60206896551724, 20.826206896551724, 20.55034482758621, 18.981379310344828, 18.429655172413796, 15.119310344827587, 16.946896551724137, 21.61931034482759, 21.446896551724137, 20.153793103448276, 17.895172413793105, 17.498620689655176, 11.550344827586208, 3.2572413793103463, 10.722758620689657, 15.119310344827587, 10.567586206896554, 13.964137931034484, 8.740000000000002, 14.946896551724137, 24.153793103448276, 22.498620689655173, 12.791724137931036, 8.395172413793105, 14.515862068965518, 15.13655172413793, 13.80896551724138, 9.240000000000002, 9.826206896551724, 7.946896551724139, 5.033103448275863, 12.705517241379312, 14.326206896551724, 16.291724137931034, 14.24, 10.653793103448278, 14.050344827586208, 12.240000000000002, 16.808965517241383, 10.550344827586208, -2.1737931034482747, -3.2944827586206884, 4.102068965517242, -0.1048275862068957, -1.3979310344827578, 6.326206896551725, 6.722758620689657, 8.533103448275863, 7.550344827586208, 7.774482758620691, 2.34344827586207, 19.964137931034482, 49.44689655172414, 71.36068965517241, 82.11931034482758, 88.01586206896552, 74.77448275862069, 41.72275862068966, 26.222758620689657, 26.860689655172415, 55.757241379310344, 129.68827586206893, 279.20551724137925, 477.6365517241379, 624.3434482758621, 596.2744827586207, 438.68827586206896, 362.61931034482757, 438.79172413793106, 476.9986206896551, 344.4468965517241, 159.70551724137928, 73.74000000000001, 61.99862068965517, 47.01586206896552, 46.84344827586207, 69.80896551724138, 108.0503448275862, 124.86068965517242, 94.74000000000001, 43.05034482758621, 16.533103448275863, 5.257241379310346, 6.171034482758621, 6.74, -3.466896551724137, -0.31172413793103315, 1.84344827586207, -2.035862068965516, -0.27724137931034365, 3.3951724137931043, 7.205517241379312, 8.671034482758621, 4.860689655172415, 4.360689655172415, 3.0675862068965527, 2.964137931034484, 9.429655172413796, 13.895172413793105, 12.446896551724139, 4.429655172413794, -1.053103448275861, 1.774482758620691, -1.0875862068965505, 2.9296551724137943, 2.791724137931036, 5.067586206896553, 6.326206896551725, -3.5186206896551715, 0.2400000000000011, 1.067586206896553, -2.6910344827586195, 3.153793103448278, 0.3434482758620705, -7.535862068965516, -2.0875862068965505, 2.481379310344829, 4.602068965517242, 7.567586206896554, -1.553103448275861, -9.242758620689655, -0.39793103448275735, 9.41241379310345, 9.636551724137933, 6.153793103448278, 0.15379310344827735, 1.1365517241379326, 1.7055172413793116, -1.4841379310344816, -3.742758620689654, -3.0186206896551715, 2.791724137931036, 6.550344827586208, -0.8117241379310327, -6.55310344827586, 0.171034482758622, 1.6882758620689668, 1.8089655172413805, -0.3289655172413781, 5.464137931034484, 8.464137931034484, 3.3951724137931047, 4.636551724137933, -2.604827586206895, -9.001379310344825, -0.6048275862068953, 4.015862068965518, 2.171034482758622, 4.205517241379312, 5.429655172413794, 6.446896551724139, 2.2744827586206906, -1.3806896551724126, -1.518620689655171, -1.4668965517241368, 2.860689655172415, 1.0158620689655184, 1.9296551724137943, 4.4124137931034495, 8.653793103448278, 4.619310344827587, 0.1537931034482769, 3.636551724137932, -2.949655172413792, -4.19103448275862, 1.6882758620689668, 0.5503448275862082, -8.62206896551724, -10.742758620689653, -7.432413793103446, -3.8462068965517227, -4.139310344827585, -1.7772413793103434, -0.5531034482758608, -2.966896551724137, 1.4986206896551735, 0.7917241379310356, -2.8634482758620674, 4.636551724137933, 4.929655172413795, 0.7055172413793116, -0.6910344827586195, -2.6393103448275848, -1.9668965517241366, 0.06758620689655315, 2.688275862068967, 2.188275862068967, 4.308965517241381, 3.8262068965517253, -5.346206896551722, -7.363448275862067, 1.3089655172413805, -1.8979310344827574, -8.846206896551724, -2.2255172413793094, 1.34344827586207, -2.9841379310344816, 1.6020689655172426, 5.515862068965518, 3.6193103448275874, -1.6393103448275852, -4.12206896551724, 0.5331034482758633]
  out "Off-Line  Bin Readings":dbl[](array[numeric])=[1504.0, 1660.0, 1829.0, 1962.0, 2184.0, 2245.0, 2446.0, 2596.0, 2676.0, 2741.0, 2803.0, 2831.0, 2987.0, 3133.0, 3087.0, 3213.0, 3306.0, 3523.0, 3752.0, 4129.0, 4474.0, 4331.0, 4066.0, 3708.0, 3737.0, 3631.0, 3740.0, 4337.0, 4328.0, 3276.0, 2325.0, 1501.0, 1323.0, 1338.0, 1254.0, 1350.0, 1246.0, 1283.0, 1265.0, 1252.0, 1318.0, 1292.0, 1255.0, 1278.0, 1301.0, 1288.0, 1316.0, 1253.0, 1271.0, 1220.0, 1216.0, 1239.0, 1167.0, 1176.0, 1320.0, 1097.0, 1206.0, 1216.0, 1188.0, 1188.0, 1214.0, 1228.0, 1233.0, 1186.0, 1241.0, 1239.0, 1207.0, 1169.0, 1142.0, 1186.0, 1176.0, 1202.0, 1209.0, 1151.0, 1132.0, 1241.0, 1166.0, 1258.0, 1185.0, 1126.0, 1204.0, 1133.0, 1211.0, 1182.0, 1146.0, 1145.0, 1165.0, 1219.0, 1155.0, 1178.0, 1196.0, 1156.0, 1186.0, 1189.0, 1174.0, 1083.0, 1132.0, 1160.0, 1162.0, 1177.0, 1238.0, 1124.0, 1197.0, 1168.0, 1161.0, 1090.0, 1174.0, 1244.0, 1219.0, 1205.0, 1176.0, 1119.0, 1166.0, 1135.0, 1190.0, 1126.0, 1130.0, 1175.0, 1094.0, 1088.0, 1177.0, 1139.0, 1140.0, 1194.0, 1081.0, 1168.0, 1197.0, 1239.0, 1179.0, 1214.0, 1225.0, 1217.0, 1214.0, 1166.0, 1174.0, 1241.0, 1284.0, 1530.0, 1768.0, 1769.0, 1668.0, 1395.0, 1455.0, 1474.0, 1526.0, 1419.0, 1149.0, 1175.0, 1184.0, 1210.0, 1308.0, 1299.0, 1287.0, 1277.0, 1198.0, 1122.0, 1152.0, 1142.0, 1181.0, 1150.0, 1190.0, 1118.0, 1165.0, 1137.0, 1178.0, 1103.0, 1156.0, 1197.0, 1206.0, 1142.0, 1121.0, 1160.0, 1225.0, 1128.0, 1183.0, 1138.0, 1118.0, 1107.0, 1055.0, 1142.0, 1084.0, 1129.0, 1156.0, 1151.0, 1195.0, 1172.0, 1139.0, 1208.0, 1245.0, 1220.0, 1186.0, 1175.0, 1164.0, 1205.0, 1177.0, 1103.0, 1224.0, 1217.0, 1108.0, 1194.0, 1171.0, 1106.0, 1167.0, 1152.0, 1156.0, 1165.0, 1153.0, 1183.0, 1169.0, 1219.0, 1177.0, 1158.0, 1155.0, 1148.0, 1166.0, 1220.0, 1152.0, 1191.0, 1145.0, 1115.0, 1213.0, 1174.0, 1099.0, 1158.0, 1148.0, 1151.0, 1180.0, 1209.0, 1143.0, 1127.0, 1152.0, 1170.0, 1117.0, 1141.0, 1163.0, 1134.0, 1198.0, 1207.0, 1137.0, 1148.0, 1145.0, 1135.0, 1141.0, 1153.0, 1187.0, 1135.0, 1157.0, 1215.0, 1120.0, 1171.0, 1176.0, 1140.0, 1106.0, 1143.0, 1158.0, 1194.0, 1123.0, 1186.0, 1166.0, 1145.0, 1133.0, 1127.0, 1180.0, 1192.0, 1171.0, 1112.0, 1203.0, 1111.0, 1122.0, 1185.0, 1203.0, 1199.0, 1175.0, 1167.0, 1169.0, 1185.0, 1163.0, 1097.0, 1183.0]
  out "Off-Line Smoothed":dbl[](array[numeric])=[402.3185106382979, 557.0631914893618, 725.1855319148935, 878.8663829787234, 1002.5312765957448, 1113.4568085106384, 1227.5153191489362, 1335.5206382978724, 1428.6748936170216, 1525.6695744680856, 1632.0259574468087, 1731.919574468085, 1824.9355319148935, 1918.3929787234044, 2017.281276595745, 2146.4355319148945, 2325.4142553191496, 2513.4036170212776, 2697.8982978723416, 2856.05255319149, 2928.5685106382975, 2926.031276595744, 2928.313191489361, 2916.4248936170206, 2833.892978723404, 2718.754680851064, 2531.9674468085113, 2203.4674468085104, 1726.4195744680849, 1108.8025531914896, 528.5738297872341, 227.91425531914888, 158.9089361702127, 150.83446808510632, 137.95680851063824, 119.7334042553191, 111.0046808510638, 102.96212765957445, 96.61638297872338, 99.791914893617, 96.39297872340421, 88.15893617021271, 86.79191489361698, 90.41957446808507, 95.83446808510638, 97.95148936170212, 91.56851063829785, 81.7706382978723, 72.15361702127657, 65.77063829787232, 63.85574468085103, 58.759999999999955, 54.41425531914889, 50.24936170212763, 46.92489361702126, 46.39829787234041, 47.83446808510636, 47.06851063829786, 42.42489361702127, 38.180212765957435, 40.05255319148935, 40.627021276595734, 36.24404255319148, 33.935531914893616, 34.38234042553191, 37.21744680851063, 37.329148936170206, 34.38765957446808, 32.01, 30.786595744680845, 28.00468085106382, 23.18021276595744, 24.32914893617021, 25.6163829787234, 22.95148936170212, 20.142978723404248, 19.329148936170206, 19.472765957446803, 20.786595744680845, 18.611063829787227, 19.05787234042553, 22.994042553191488, 20.818510638297866, 19.212127659574463, 20.20680851063829, 18.568510638297866, 17.27063829787233, 15.573829787234036, 13.382340425531908, 12.744042553191484, 9.834468085106376, 10.483404255319142, 12.690851063829781, 15.627021276595737, 18.882340425531908, 18.70680851063829, 15.105744680851057, 14.818510638297866, 16.786595744680845, 15.552553191489356, 13.775957446808505, 12.892978723404248, 13.18021276595744, 10.898297872340418, 6.786595744680844, 6.759999999999994, 8.749361702127654, 11.259999999999994, 11.823829787234036, 10.371702127659567, 10.898297872340418, 7.967446808510632, 10.515319148936165, 11.972765957446803, 6.690851063829781, 3.8663829787233976, 6.0472340425531845, 7.967446808510632, 6.403617021276589, 7.371702127659567, 9.020638297872335, 6.0897872340425465, 2.031276595744674, 4.967446808510632, 11.68553191489361, 35.57382978723402, 61.898297872340386, 72.81319148936166, 72.27063829787231, 68.6482978723404, 56.451489361702095, 33.97808510638296, 25.44617021276595, 36.1323404255319, 75.02063829787232, 157.0578723404255, 298.9142553191489, 484.4248936170212, 646.3557446808511, 640.3929787234044, 448.90361702127655, 312.8131914893616, 358.79723404255316, 413.65893617021277, 320.24404255319143, 159.11106382978716, 75.0206382978723, 64.71744680851062, 60.717446808510616, 54.31319148936167, 58.07914893617017, 90.24404255319143, 114.56319148936167, 91.2227659574468, 43.86106382978722, 12.355744680851057, 5.142978723404249, 5.940851063829781, 6.398297872340419, 3.1057446808510574, 2.2440425531914827, 1.877021276595738, -0.9793617021276663, 0.6163829787233974, 0.8823404255319082, -0.21340425531915552, 0.6695744680850997, 2.2121276595744614, 4.228085106382972, 0.7919148936170146, 1.5099999999999933, 4.579148936170206, 4.978085106382972, 7.217446808510632, 4.834468085106376, 1.9993617021276529, 2.573829787234036, 1.025957446808504, 2.520638297872334, 3.403617021276589, 2.531276595744674, 2.43021276595744, -0.11765957446809178, -0.6336170212766025, -0.3357446808510705, 0.5365957446808444, 1.829148936170206, -0.059148936170219546, -0.9846808510638365, 0.7280851063829721, 4.217446808510632, 3.5791489361702062, 2.2599999999999936, -0.5644680851063897, -3.979361702127666, -1.2612765957446876, 0.16425531914892952, 1.504680851063823, 4.994042553191482, 4.515319148936164, 6.334468085106376, 3.5951063829787167, -2.479361702127666, -2.202765957446815, -0.21340425531915552, 2.020638297872334, 1.8238297872340359, 0.08446808510637638, -0.7027659574468151, -0.47404255319149613, -0.8995744680851131, 3.025957446808504, 3.653617021276589, 2.781276595744674, 3.1642553191489293, 2.0791489361702062, 1.7334042553191422, -0.17085106382979398, -4.351702127659581, 0.17489361702127004, 3.073829787234036, -2.9208510638297938, -2.5059574468085173, 1.9887234042553126, 5.478085106382972, 4.898297872340419, 1.6642553191489295, 1.3876595744680784, -1.9634042553191555, -3.8942553191489426, -2.6761702127659643, -0.24000000000000687, 1.5312765957446741, 2.0365957446808443, 0.653617021276589, -2.091063829787241, 1.254680851063823, 2.3929787234042488, 2.9993617021276533, 4.701489361702121, 2.398297872340419, -2.2878723404255386, -4.335744680851071, -5.5378723404255386, -4.154893617021283, 1.7174468085106314, 2.2865957446808443, -2.729361702127666, -2.899574468085113, -2.9368085106383046, -2.6602127659574535, -1.8995744680851132, 2.6961702127659506, 3.871702127659568, 0.8610638297872274, 3.3823404255319085, 1.7121276595744614, -1.1282978723404322, -1.8995744680851132, 0.3610638297872274, 1.7812765957446741, 2.8663829787233976, 3.648297872340419, 0.7334042553191423, -1.2027659574468152, -0.35170212765958114, -3.101702127659581, -6.979361702127667, -0.9155319148936241, 2.6802127659574397, 0.2812765957446742, 1.3397872340425465, 1.2812765957446741, 0.7493617021276529, -3.5538297872340494, -5.638936170212773, -0.5697872340425598]
  out "On-Line  Smoothed":dbl[](array[numeric])=[357.9972340425532, 471.49723404255315, 579.4068085106383, 661.3217021276596, 717.0451063829787, 762.1089361702127, 801.6355319148936, 828.7472340425531, 847.896170212766, 861.5451063829787, 874.0397872340426, 880.5504255319149, 883.646170212766, 891.8110638297873, 900.7525531914894, 918.7206382978725, 945.9068085106385, 978.3536170212768, 1017.4706382978725, 1040.4493617021278, 1027.608936170213, 994.9972340425533, 963.2951063829789, 920.6302127659576, 865.3217021276596, 805.7153191489361, 729.1461702127658, 616.6408510638296, 470.07170212765953, 299.646170212766, 141.87489361702126, 60.64085106382981, 39.36425531914896, 34.587659574468105, 33.710000000000015, 32.566382978723425, 27.731276595744696, 21.23659574468086, 23.18872340425533, 21.779148936170223, 18.699361702127668, 20.725957446808515, 24.725957446808515, 25.33234042553192, 19.656808510638307, 14.199361702127668, 14.667446808510647, 16.614255319148945, 15.02914893617022, 14.970638297872348, 15.03446808510639, 13.56638297872341, 12.82170212765958, 12.119574468085112, 8.103617021276602, 5.8110638297872415, 4.736595744680859, 4.592978723404263, 6.167446808510645, 6.6461702127659645, 8.928085106382987, 10.06638297872341, 7.369574468085114, 3.880212765957454, 2.0557446808510713, 6.662127659574475, 7.119574468085114, 6.087659574468093, 6.997234042553199, 5.406808510638305, 4.608936170212774, 2.662127659574476, 1.8482978723404329, 2.486595744680858, 3.630212765957454, 3.3961702127659645, 5.4387234042553265, 6.694042553191497, 7.013191489361709, 7.247234042553199, 4.348297872340433, 4.247234042553199, 5.316382978723412, 1.0504255319149007, 2.4227659574468157, 3.348297872340433, 2.997234042553199, 5.321702127659582, 5.353617021276603, 4.215319148936177, 2.5131914893617093, 3.9440425531914967, 1.5982978723404326, 4.263191489361709, 1.2631914893617098, -1.210212765957439, 4.039787234042561, 2.880212765957454, 3.874893617021284, 2.1887234042553265, -0.9548936170212693, 1.6514893617021351, 2.4653191489361777, -2.6836170212765884, 0.14617021276596454, 2.327021276595752, 0.624893617021284, 5.140851063829794, 2.6408510638297944, 0.41744680851064575, 3.422765957446816, 1.2791489361702202, -1.997446808510631, -0.4442553191489287, 0.7738297872340499, 3.0451063829787306, 3.077021276595752, 4.135531914893624, 6.05574468085107, 2.2419148936170283, -0.16234042553190758, -2.3112765957446735, -0.9123404255319076, 2.124893617021284, 3.757872340425539, 6.433404255319156, 11.975957446808518, 17.151489361702133, 16.08234042553192, 13.02914893617022, 11.06106382978724, 9.651489361702135, 4.741914893617029, 1.9174468085106458, 12.27382978723405, 33.332340425531925, 64.8748936170213, 104.4972340425532, 138.31106382978723, 140.1195744680851, 99.08234042553192, 70.2844680851064, 78.2685106382979, 87.72595744680854, 68.24191489361704, 33.773829787234064, 12.497234042553199, 11.646170212765965, 18.358936170212772, 15.704680851063838, 13.460000000000008, 20.32170212765958, 20.678085106382987, 11.635531914893626, 5.603617021276603, 1.7685106382978797, 2.5344680851063903, 1.678085106382986, -1.0346808510638226, -1.2102127659574395, 2.725957446808518, 3.7365957446808586, -0.1570212765957374, -1.4282978723404183, -2.0825531914893545, -2.417659574468078, -2.029361702127652, -2.289999999999993, 0.5982978723404329, 1.9706382978723478, -0.21021276595743943, 0.19404255319149677, 2.5185106382978795, -0.29531914893616285, -1.252765957446801, 1.8589361702127734, -1.3751063829787162, -2.3644680851063757, -0.7208510638297799, -0.9708510638297799, -3.0559574468085033, -3.7580851063829717, -3.125106382978716, -3.3059574468085033, -0.5559574468085033, 0.6461702127659648, -1.5772340425531841, -4.045319148936163, -3.492127659574461, 0.16744680851064553, 1.752553191489369, -0.9442553191489287, -1.7421276595744608, 0.6993617021276669, 2.52914893617022, 2.795106382978731, 2.0929787234042627, 1.6408510638297946, 2.460000000000007, 0.26319148936170933, -1.7793617021276522, -1.7580851063829712, -3.4708510638297803, -0.6144680851063757, -1.125106382978716, -4.9389361702127585, -4.800638297872332, -3.258085106382971, -3.571914893617014, -2.162340425531908, -1.1091489361702056, -2.0665957446808436, 1.5291489361702202, 2.4387234042553265, 2.5610638297872415, 2.619574468085114, -0.1942553191489289, -1.8165957446808436, -3.5134042553191414, -4.758085106382971, -4.337872340425525, -4.135744680851056, -0.7634042553191416, -4.247446808510631, -3.821914893617014, 1.5557446808510713, -2.768723404255312, -5.19425531914893, -0.09851063829786533, 1.5504255319149007, -3.646382978723397, -0.5027659574468011, 0.5025531914893693, -1.8112765957446735, 0.27382978723404994, 0.6142553191489435, -0.1357446808510565, -4.194255319148929, -0.332553191489354, 1.039787234042561, -2.8644680851063753, -3.082553191489354, 0.2791489361702202, 4.390851063829794, 2.5717021276595817, 0.6355319148936244, 0.2951063829787308, -1.6623404255319074, -3.23148936170212, -1.9708510638297798, -0.008085106382971441, 0.5397872340425605, -1.5453191489361628, -3.795319148936163, -0.6410638297872269, 5.369574468085114, 3.880212765957454, -0.3857446808510565, -2.029361702127652, 0.39617021276596476, 4.949361702127667, 4.055744680851071, -0.8272340425531842, -2.401702127659567, 2.3376595744680926, 3.577021276595752, 2.082340425531922, -0.07191489361701398, -2.0665957446808436, -0.9602127659574394, -2.1144680851063757, -3.8112765957446735, -3.125106382978716, 0.9546808510638373, -0.3591489361702054, -1.6304255319148864, -1.71553191489361]
  out "On-Line Bin Readings":dbl[](array[numeric])=[1364.0, 1534.0, 1741.0, 1806.0, 1907.0, 1964.0, 2053.0, 2043.0, 1951.0, 2053.0, 1967.0, 2068.0, 2013.0, 2015.0, 2057.0, 2099.0, 2031.0, 2134.0, 2150.0, 2217.0, 2422.0, 2303.0, 2083.0, 1990.0, 1871.0, 1869.0, 1886.0, 2046.0, 1939.0, 1731.0, 1473.0, 1202.0, 1163.0, 1173.0, 1220.0, 1228.0, 1151.0, 1164.0, 1232.0, 1224.0, 1179.0, 1152.0, 1185.0, 1172.0, 1219.0, 1158.0, 1168.0, 1204.0, 1162.0, 1200.0, 1139.0, 1125.0, 1169.0, 1180.0, 1175.0, 1143.0, 1155.0, 1207.0, 1149.0, 1161.0, 1151.0, 1168.0, 1161.0, 1170.0, 1124.0, 1083.0, 1186.0, 1124.0, 1217.0, 1181.0, 1191.0, 1170.0, 1125.0, 1091.0, 1164.0, 1101.0, 1173.0, 1145.0, 1180.0, 1144.0, 1177.0, 1134.0, 1244.0, 1136.0, 1190.0, 1157.0, 1136.0, 1194.0, 1166.0, 1131.0, 1148.0, 1167.0, 1134.0, 1108.0, 1126.0, 1150.0, 1153.0, 1171.0, 1189.0, 1159.0, 1213.0, 1210.0, 1117.0, 1189.0, 1160.0, 1164.0, 1184.0, 1121.0, 1185.0, 1142.0, 1073.0, 1182.0, 1124.0, 1157.0, 1134.0, 1075.0, 1145.0, 1157.0, 1141.0, 1180.0, 1096.0, 1149.0, 1096.0, 1187.0, 1142.0, 1204.0, 1142.0, 1156.0, 1147.0, 1156.0, 1218.0, 1155.0, 1196.0, 1143.0, 1118.0, 1145.0, 1207.0, 1198.0, 1268.0, 1343.0, 1279.0, 1249.0, 1272.0, 1198.0, 1238.0, 1265.0, 1140.0, 1109.0, 1162.0, 1150.0, 1123.0, 1209.0, 1189.0, 1153.0, 1157.0, 1171.0, 1170.0, 1116.0, 1183.0, 1143.0, 1086.0, 1144.0, 1163.0, 1134.0, 1184.0, 1169.0, 1198.0, 1101.0, 1134.0, 1157.0, 1148.0, 1056.0, 1087.0, 1138.0, 1153.0, 1278.0, 1163.0, 1253.0, 1186.0, 1233.0, 1124.0, 1107.0, 1167.0, 1206.0, 1157.0, 1094.0, 1155.0, 1227.0, 1088.0, 1204.0, 1164.0, 1155.0, 1185.0, 1177.0, 1149.0, 1191.0, 1151.0, 1155.0, 1172.0, 1220.0, 1176.0, 1155.0, 1169.0, 1162.0, 1146.0, 1111.0, 1194.0, 1194.0, 1125.0, 1144.0, 1183.0, 1156.0, 1181.0, 1169.0, 1150.0, 1142.0, 1201.0, 1114.0, 1171.0, 1123.0, 1173.0, 1231.0, 1172.0, 1206.0, 1190.0, 1127.0, 1183.0, 1126.0, 1100.0, 1226.0, 1144.0, 1127.0, 1141.0, 1109.0, 1191.0, 1121.0, 1142.0, 1198.0, 1161.0, 1179.0, 1152.0, 1175.0, 1100.0, 1087.0, 1182.0, 1185.0, 1145.0, 1123.0, 1137.0, 1137.0, 1191.0, 1142.0, 1158.0, 1159.0, 1159.0, 1185.0, 1067.0, 1221.0, 1171.0, 1166.0, 1128.0, 1156.0, 1126.0, 1103.0, 1126.0, 1160.0, 1155.0, 1206.0, 1187.0, 1218.0, 1226.0, 1091.0, 1145.0, 1190.0, 1183.0, 1182.0, 1182.0, 1175.0, 1123.0]
  out "Range Corrected Altitude Array":dbl[](array[numeric])=[5625.0, 22500.0, 50625.0, 90000.0, 140625.0, 202500.0, 275625.0, 360000.0, 455625.0, 562500.0, 680625.0, 810000.0, 950625.0, 1102500.0, 1265625.0, 1440000.0, 1625625.0, 1822500.0, 2030625.0, 2250000.0, 2480625.0, 2722500.0, 2975625.0, 3240000.0, 3515625.0, 3802500.0, 4100625.0, 4410000.0, 4730625.0, 5062500.0, 5405625.0, 5760000.0, 6125625.0, 6502500.0, 6890625.0, 7290000.0, 7700625.0, 8122500.0, 8555625.0, 9000000.0, 9455625.0, 9922500.0, 10400625.0, 10890000.0, 11390625.0, 11902500.0, 12425625.0, 12960000.0, 13505625.0, 14062500.0, 14630625.0, 15210000.0, 15800625.0, 16402500.0, 17015625.0, 17640000.0, 18275625.0, 18922500.0, 19580625.0, 20250000.0, 20930625.0, 21622500.0, 22325625.0, 23040000.0, 23765625.0, 24502500.0, 25250625.0, 26010000.0, 26780625.0, 27562500.0, 28355625.0, 29160000.0, 29975625.0, 30802500.0, 31640625.0, 32490000.0, 33350625.0, 34222500.0, 35105625.0, 36000000.0, 36905625.0, 37822500.0, 38750625.0, 39690000.0, 40640625.0, 41602500.0, 42575625.0, 43560000.0, 44555625.0, 45562500.0, 46580625.0, 47610000.0, 48650625.0, 49702500.0, 50765625.0, 51840000.0, 52925625.0, 54022500.0, 55130625.0, 56250000.0, 57380625.0, 58522500.0, 59675625.0, 60840000.0, 62015625.0, 63202500.0, 64400625.0, 65610000.0, 66830625.0, 68062500.0, 69305625.0, 70560000.0, 71825625.0, 73102500.0, 74390625.0, 75690000.0, 77000625.0, 78322500.0, 79655625.0, 81000000.0, 82355625.0, 83722500.0, 85100625.0, 86490000.0, 87890625.0, 89302500.0, 90725625.0, 92160000.0, 93605625.0, 95062500.0, 96530625.0, 98010000.0, 99500625.0, 101002500.0, 102515625.0, 104040000.0, 105575625.0, 107122500.0, 108680625.0, 110250000.0, 111830625.0, 113422500.0, 115025625.0, 116640000.0, 118265625.0, 119902500.0, 121550625.0, 123210000.0, 124880625.0, 126562500.0, 128255625.0, 129960000.0, 131675625.0, 133402500.0, 135140625.0, 136890000.0, 138650625.0, 140422500.0, 142205625.0, 144000000.0, 145805625.0, 147622500.0, 149450625.0, 151290000.0, 153140625.0, 155002500.0, 156875625.0, 158760000.0, 160655625.0, 162562500.0, 164480625.0, 166410000.0, 168350625.0, 170302500.0, 172265625.0, 174240000.0, 176225625.0, 178222500.0, 180230625.0, 182250000.0, 184280625.0, 186322500.0, 188375625.0, 190440000.0, 192515625.0, 194602500.0, 196700625.0, 198810000.0, 200930625.0, 203062500.0, 205205625.0, 207360000.0, 209525625.0, 211702500.0, 213890625.0, 216090000.0, 218300625.0, 220522500.0, 222755625.0, 225000000.0, 227255625.0, 229522500.0, 231800625.0, 234090000.0, 236390625.0, 238702500.0, 241025625.0, 243360000.0, 245705625.0, 248062500.0, 250430625.0, 252810000.0, 255200625.0, 257602500.0, 260015625.0, 262440000.0, 264875625.0, 267322500.0, 269780625.0, 272250000.0, 274730625.0, 277222500.0, 279725625.0, 282240000.0, 284765625.0, 287302500.0, 289850625.0, 292410000.0, 294980625.0, 297562500.0, 300155625.0, 302760000.0, 305375625.0, 308002500.0, 310640625.0, 313290000.0, 315950625.0, 318622500.0, 321305625.0, 324000000.0, 326705625.0, 329422500.0, 332150625.0, 334890000.0, 337640625.0, 340402500.0, 343175625.0, 345960000.0, 348755625.0, 351562500.0, 354380625.0, 357210000.0, 360050625.0, 362902500.0, 365765625.0, 368640000.0, 371525625.0, 374422500.0, 377330625.0, 380250000.0, 383180625.0, 386122500.0, 389075625.0, 392040000.0, 395015625.0, 398002500.0, 401000625.0, 404010000.0, 407030625.0, 410062500.0, 413105625.0, 416160000.0, 419225625.0, 422302500.0, 425390625.0, 428490000.0, 431600625.0, 434722500.0, 437855625.0, 441000000.0]
  out "Altitude Array (km)":dbl[](array[numeric])=[0.075, 0.15, 0.22499999999999998, 0.3, 0.375, 0.45, 0.5249999999999999, 0.6, 0.6749999999999999, 0.7499999999999999, 0.825, 0.8999999999999999, 0.9749999999999999, 1.05, 1.125, 1.2, 1.275, 1.3499999999999999, 1.4249999999999998, 1.5, 1.575, 1.65, 1.7249999999999999, 1.7999999999999998, 1.8749999999999998, 1.95, 2.025, 2.1, 2.1750000000000003, 2.25, 2.325, 2.4, 2.475, 2.5500000000000003, 2.625, 2.7, 2.775, 2.85, 2.9250000000000003, 3.0, 3.075, 3.15, 3.225, 3.3000000000000003, 3.375, 3.45, 3.525, 3.6, 3.675, 3.75, 3.825, 3.9, 3.975, 4.05, 4.125, 4.2, 4.275, 4.35, 4.425, 4.5, 4.575, 4.65, 4.725, 4.8, 4.875, 4.95, 5.025, 5.1, 5.175, 5.25, 5.325, 5.4, 5.475, 5.55, 5.625, 5.7, 5.775, 5.85, 5.925, 6.0, 6.075, 6.15, 6.225, 6.3, 6.375, 6.45, 6.525, 6.6, 6.675, 6.75, 6.825, 6.9, 6.975, 7.05, 7.125, 7.2, 7.2749999999999995, 7.35, 7.425, 7.5, 7.575, 7.6499999999999995, 7.725, 7.8, 7.875, 7.95, 8.024999999999999, 8.1, 8.174999999999999, 8.249999999999998, 8.325, 8.399999999999999, 8.475, 8.549999999999999, 8.624999999999998, 8.7, 8.774999999999999, 8.85, 8.924999999999999, 8.999999999999998, 9.075, 9.149999999999999, 9.225, 9.299999999999999, 9.374999999999998, 9.45, 9.524999999999999, 9.6, 9.674999999999999, 9.749999999999998, 9.825, 9.899999999999999, 9.975, 10.049999999999999, 10.124999999999998, 10.2, 10.274999999999999, 10.35, 10.424999999999999, 10.499999999999998, 10.575, 10.649999999999999, 10.725, 10.799999999999999, 10.874999999999998, 10.95, 11.024999999999999, 11.1, 11.174999999999999, 11.249999999999998, 11.325, 11.399999999999999, 11.475, 11.549999999999999, 11.624999999999998, 11.7, 11.774999999999999, 11.85, 11.924999999999999, 11.999999999999998, 12.075, 12.149999999999999, 12.225, 12.299999999999999, 12.374999999999998, 12.45, 12.524999999999999, 12.6, 12.674999999999999, 12.749999999999998, 12.825, 12.899999999999999, 12.975, 13.049999999999999, 13.124999999999998, 13.2, 13.274999999999999, 13.35, 13.424999999999999, 13.499999999999998, 13.575, 13.649999999999999, 13.725, 13.799999999999999, 13.874999999999998, 13.95, 14.024999999999999, 14.1, 14.174999999999999, 14.249999999999998, 14.325, 14.399999999999999, 14.474999999999998, 14.549999999999999, 14.624999999999998, 14.7, 14.774999999999999, 14.849999999999998, 14.924999999999999, 14.999999999999998, 15.075, 15.149999999999999, 15.224999999999998, 15.299999999999999, 15.374999999999998, 15.45, 15.524999999999999, 15.599999999999998, 15.674999999999999, 15.749999999999998, 15.825, 15.899999999999999, 15.974999999999998, 16.05, 16.125, 16.2, 16.275, 16.349999999999998, 16.424999999999997, 16.5, 16.575, 16.65, 16.724999999999998, 16.799999999999997, 16.875, 16.95, 17.025, 17.099999999999998, 17.174999999999997, 17.25, 17.325, 17.4, 17.474999999999998, 17.549999999999997, 17.625, 17.7, 17.775, 17.849999999999998, 17.924999999999997, 18.0, 18.075, 18.15, 18.224999999999998, 18.299999999999997, 18.375, 18.45, 18.525, 18.599999999999998, 18.674999999999997, 18.75, 18.825, 18.9, 18.974999999999998, 19.049999999999997, 19.125, 19.2, 19.275, 19.349999999999998, 19.424999999999997, 19.5, 19.575, 19.65, 19.724999999999998, 19.799999999999997, 19.875, 19.95, 20.025, 20.099999999999998, 20.174999999999997, 20.25, 20.325, 20.4, 20.474999999999998, 20.549999999999997, 20.625, 20.7, 20.775, 20.849999999999998, 20.924999999999997, 21.0]
  in  "Instrument Control":T4(tab)
  out "Readings":T5={"OnLineTEC"=19.6067448, "OnLineLD"=0.150576174, "OffLineTEC"=18.6642399, "OffLineLD"=0.149945319, "EtalonTEC"=28.1419601, "TSOA-TEC"=19.9770756, "Pro8000"=TRUE, "OnLine TEC"=TRUE, "OnLine LD"=TRUE, "OffLine TEC"=TRUE, "OffLine LD"=TRUE, "Etalon TEC"=TRUE, "TSOA TEC"=TRUE} {"OffLineLD" format="%.4g"; "OnLineLD" format="%.4g"; "TSOA-TEC" format="%.3g"; "EtalonTEC" format="%.3g"; "OffLineTEC" format="%.3g"; "OnLineTEC" format="%.3g"}
  in  "Settings":T6={"Module"=enum."On Line TEC", "OnLineTEC"=19.601080000000486, "OnLineLD"=0.15, "OffLineTEC"=18.663800000000133, "OffLineLD"=0.15, "EtalonTEC"=28.15, "TSOA-TEC"=20.0} {"OffLineLD" min=0.0 max=0.175 step=0.001 format="%.3p"; "OnLineLD" min=0.0 max=0.175 step=0.001 format="%.3p"; "TSOA-TEC" format="%.2g"; "EtalonTEC" format="%.2g"; "OffLineTEC" min=0.0 max=30.0 step=0.1 format="%.3g"; "OnLineTEC" min=0.0 max=30.0 step=0.1 format="%.3g"}
  in  "Pulse B Polarity":enum32{"Low", "High"}(ring)=enum."High"
  in  "Pulse A Delay(ns)":u32=1040 min=80 max=327600
  in  "Pulse B Delay(ns)":u32=170000 min=80 max=327600 step=1
  in  "Accumulation Delay(ns)":u32=10 min=10 max=1270 step=1
  in  "Sync Pulse Polarity":enum32{"Low", "High"}(ring)=enum."High"
  in  "Pulse A Polarity":enum32{"Low", "High"}(ring)=enum."High"
  in  "Number of Bins":u32=280 min=2 max=4095 step=1
  in  "Number of Accumulates":u32=10000 min=1 max=32767 step=1
  in  "Time Resolution Per Bin(ns)":u32=500 min=5 max=1063 step=1
  out "WM Switch":bool
  in  "Cancel online":bool
  in  "Cancel Offline":bool
  in  "Lambda On Set (nm)":dbl=828.199 format="%.5f"
  out "Lambda On Read (nm)":dbl=828.1989809259087 format="%.5f"
  out "Lambda Off Read (nm)":dbl=828.2985857197202 format="%.5f"
  in  "Lambda Off Set (nm)":dbl=828.29865 format="%#.5f"
  in  "Bristol In":i32=5
  out "Bristol Out":i32=1
  in  "Online_Tol":dbl=5e-05 format="%#_15g"
  in  "Offline_Tol":dbl=0.0001 format="%#_15g"
  out "Wavelength Lock Online":bool=TRUE
  out "Wavelength Lock Offline":bool=TRUE
  out "WL Difference":dbl=-1.9074091255788517e-05 format="%_7g"
  out "WL Difference off":dbl=-6.42802797301556e-05 format="%_7g"
  in  "calculate absorption cross sections":bool
  in  "Smoothing Range":dbl=150.0
  in  "Total DIAL Integration Time (Minutes)":i32=3
  in  "Data Reads (number of loops)":i32=1
  in  "Total Aerosol Integration Time (Minutes)":dbl=0.5
  in  "Scalar Wait Time (disabled)":u32
  out "Smoothed Bins":dbl=2.0
  in  "Ophir PM On/Off":bool=TRUE
  out "OphirPM":T7={"Ophir-Ref"=refnum, "Ophir-Device"=1000, "Ophir-Channel"=0}
  out "Average Diode Power":dbl(knob)=0.00174 scale=0.0..0.002 scale format="%.1p"
  out "Ophir Samples":i32=30
  in  "Switch Comm Port":refnum<visa-resource-name>="COM3"
  out "FF_On_Ref":refnum<file>
  out "FF_On_Ptr":i64=215072 format="%.2p"
  out "FF_Off_Ref":refnum<file>
  out "FF_Off_Ptr":i64=215072 format="%.2p"
  out "NF_On_Ref":refnum<file>
  out "NF_On_Ptr":i64=215072 format="%.2p"
  out "NF_Off_Ref":refnum<file>
  out "NF_Off_Ptr":i64=215072 format="%.2p"
  out "DataOpen":bool=TRUE
  out "File Path_Far Field (out)":string="D:\\Micropulse_DIAL_data\\170424FF\\14"
  out "File Path_Near Field (out)":string="D:\\Micropulse_DIAL_data\\170424NF\\14"
  in  "Data File DIR (in)":string="D:\\Micropulse_DIAL_data\\"
  in  "WS_On/Off":bool=TRUE
  in  "WS visa":refnum<visa-resource-name>="Weather"
  out "TRHP":T8={"Temp C"=25.519230769230774, "RelH %"=37.15201465201466, "Press hPa"=977.3351648351648, "AbH g/m^3"=7.554945054945055}
  in  "ADAM6018 IP":string="192.168.0.165"
  out "T_bench":sgl=22.705425
  in  "Port":u16=502
  in  "IP Address":string="192.168.0.165"
  out "ID_out":refnum<k5>
  in  "bins":u32=280 min=2 max=4095 step=1
  out "y offset":u32=10
  in  "ns scale":u32=500
  # "ADAM6018"
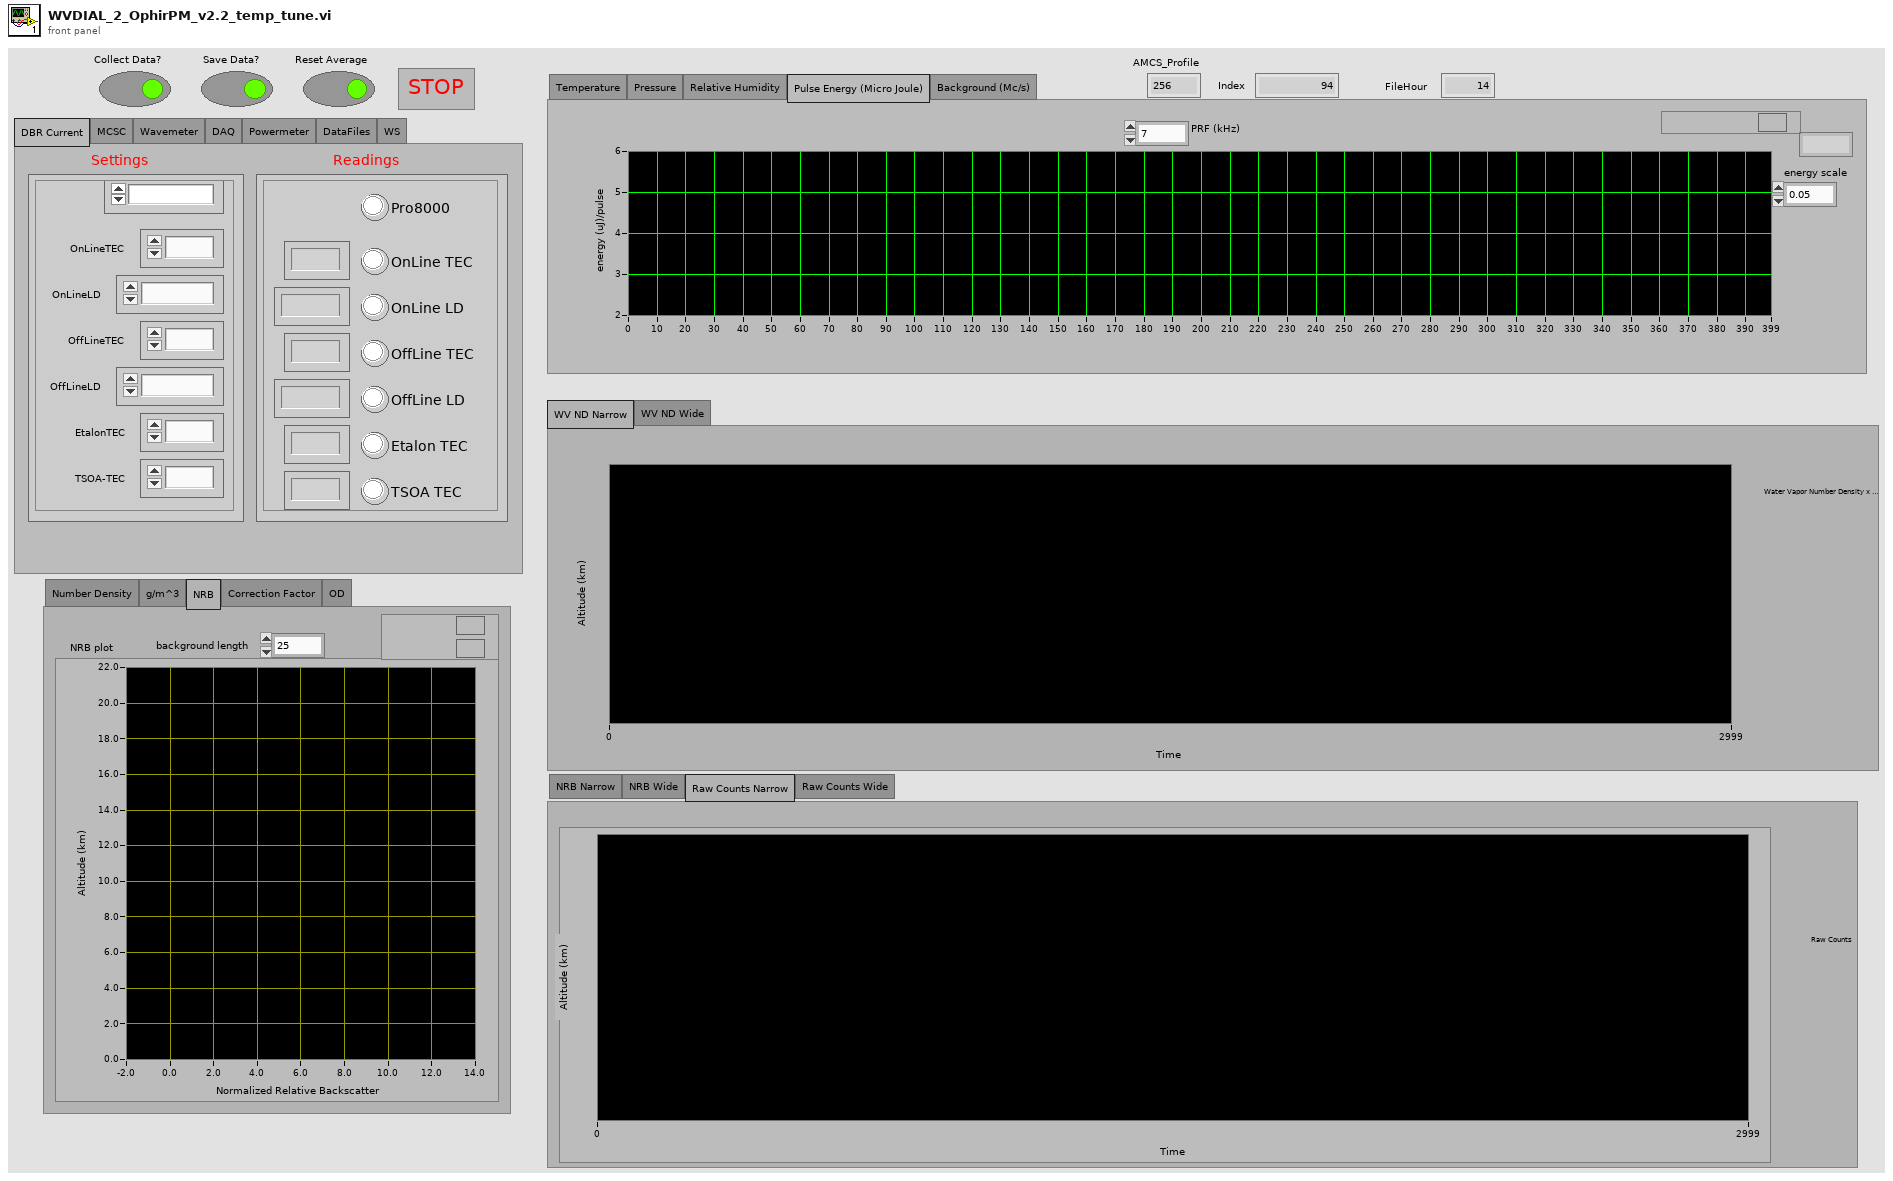
[diagram p1: front panel]
types:
  T1 = enum32{"NRB Narrow", "NRB Wide", "Raw Counts Narrow", "Raw Counts Wide"}
  T2 = enum32{"Number Density", "g/m^3", "NRB", "Correction Factor", "OD"}
  T3 = enum32{"Temperature", "Pressure", "Relative Humidity", "Pulse Energy (Micro Joule)", "Background (Mc/s)"}
  T4 = enum32{"DBR Current", "MCSC", "Wavemeter", "DAQ", "Powermeter", "DataFiles", "WS"}
  T5 = cluster{"OnLineTEC":dbl, "OnLineLD":dbl, "OffLineTEC":dbl, "OffLineLD":dbl, "EtalonTEC":dbl, "TSOA-TEC":dbl, "Pro8000":bool, "OnLine TEC":bool, "OnLine LD":bool, "OffLine TEC":bool, "OffLine LD":bool, "Etalon TEC":bool, "TSOA TEC":bool}
  T6 = cluster{"Module":enum16{"On Line TEC", "On Line LD", "Off Line TEC", "Off Line LD", "Etalon TEC", "TSOA TEC"}, "OnLineTEC":dbl, "OnLineLD":dbl, "OffLineTEC":dbl, "OffLineLD":dbl, "EtalonTEC":dbl, "TSOA-TEC":dbl}
  T7 = cluster{"Ophir-Ref":refnum<k7>, "Ophir-Device":i32, "Ophir-Channel":i32}
  T8 = cluster{"Temp C":dbl, "RelH %":dbl, "Press hPa":dbl, "AbH g/m^3":dbl}
  T9 = enum16{"Open_TL", "Close_TL", "Verify_ID", "TEC_Sensor", "SET", "READ", "ON", "OFF", "Set_Limits", "Read_Limits", "Enable_Status", "Read_Status"}
  T10 = enum16{"open", "replace", "create", "open or create", "replace or create", "replace or create with confirmation"}
  T11 = enum16{"On Line TEC", "On Line LD", "Off Line TEC", "Off Line LD", "Etalon TEC", "TSOA TEC"}
  T12 = cluster{"Temp":dbl, "RelH":dbl, "Press":dbl, "AbH":dbl}
  T13 = typedef "LVDateTimeRec.ctl" = cluster{"fractional second":dbl, "second":i32, "minute":i32, "hour":i32, "day of month":i32, "month":i32, "year":i32, "day of week":i32, "day of year":i32, "DST":i32}
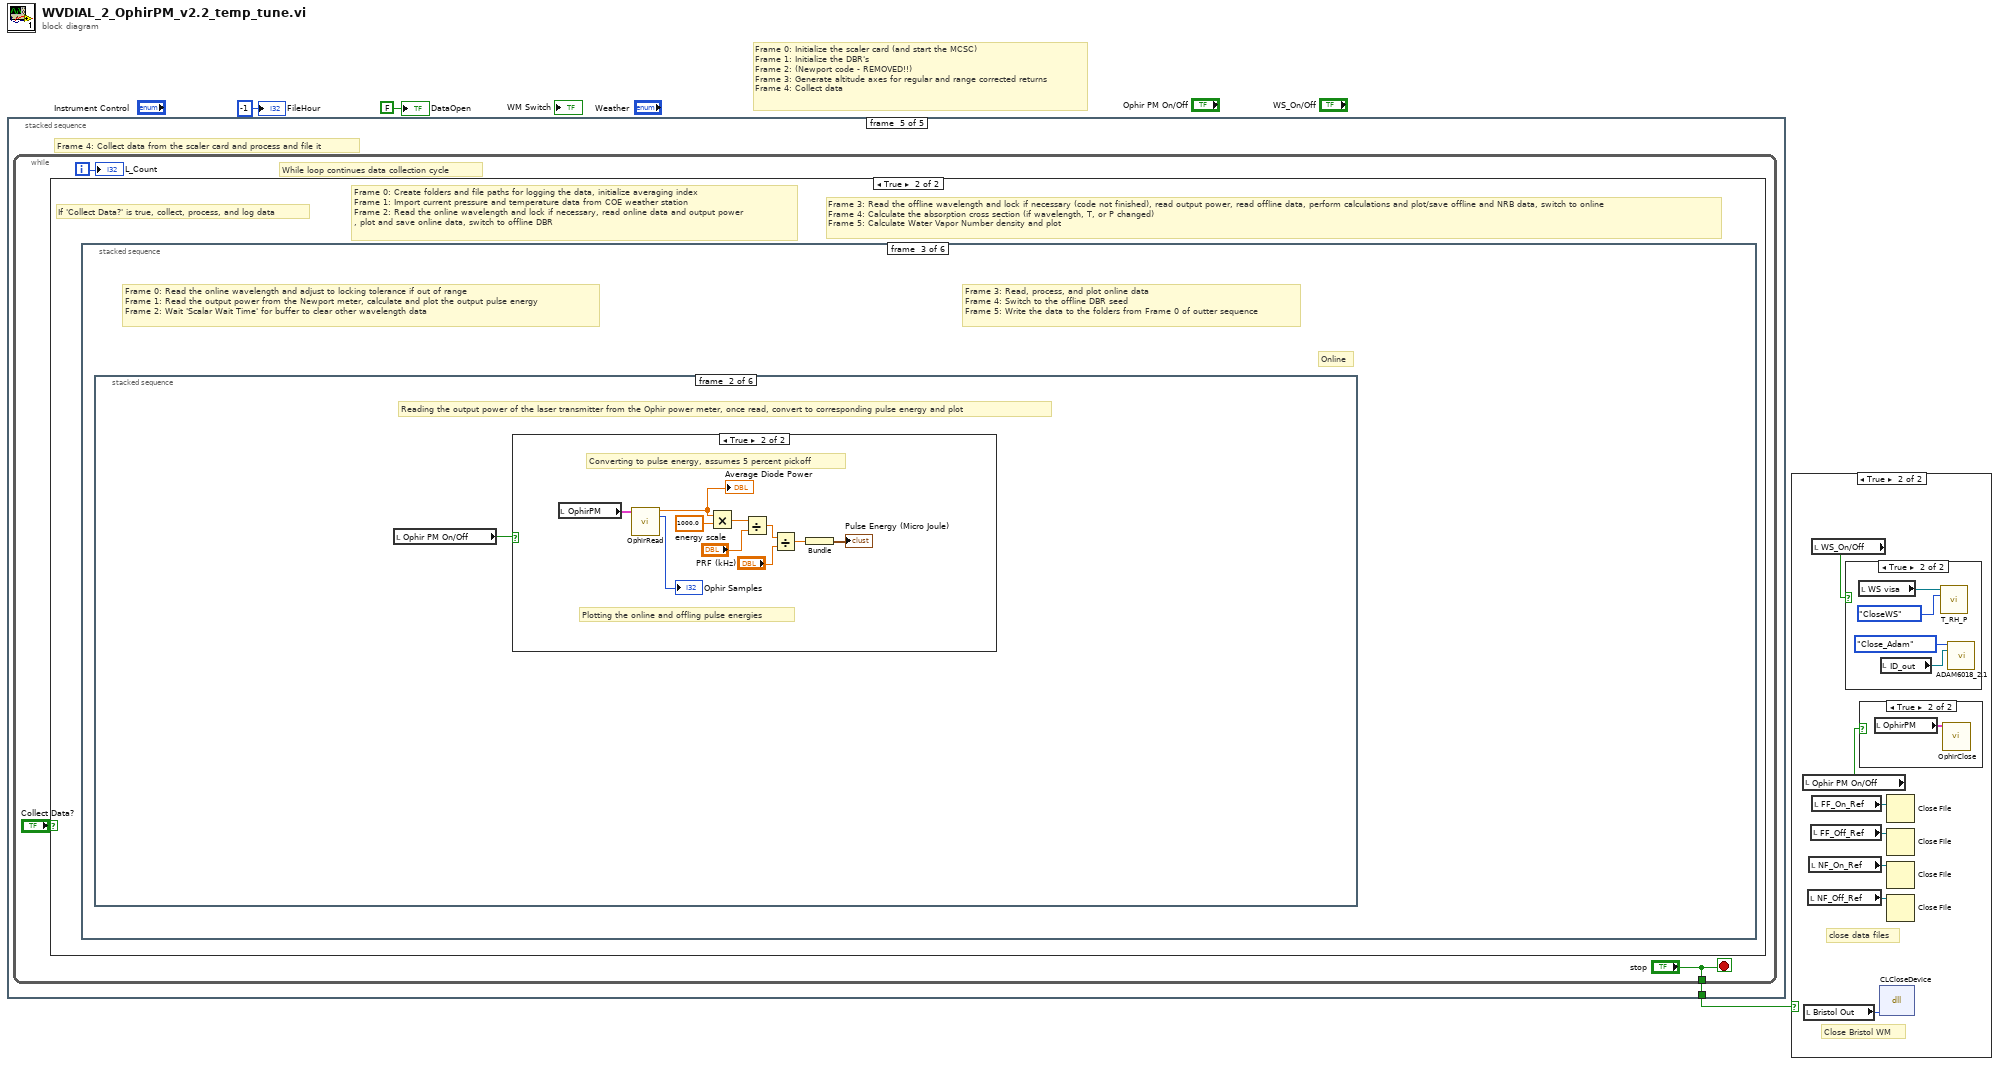
[diagram p0: block diagram]
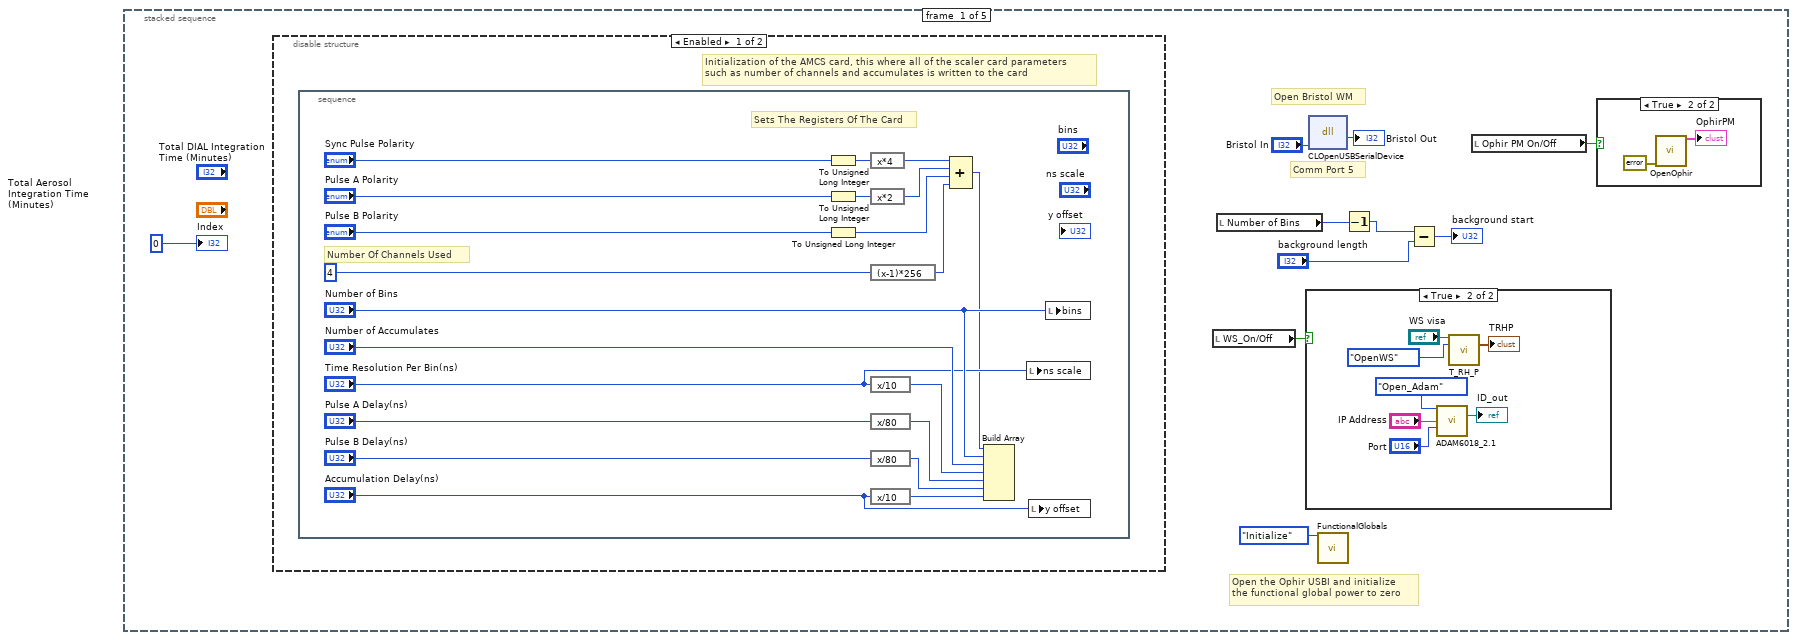
[diagram p5: hidden frame]
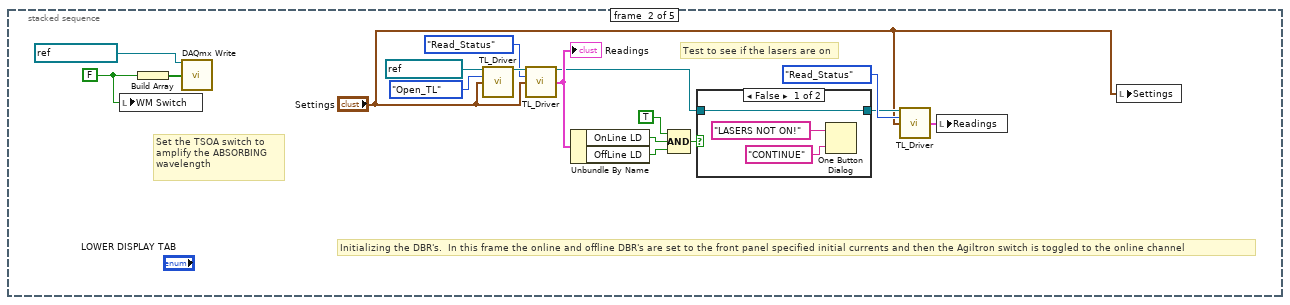
[diagram p9: hidden frame]
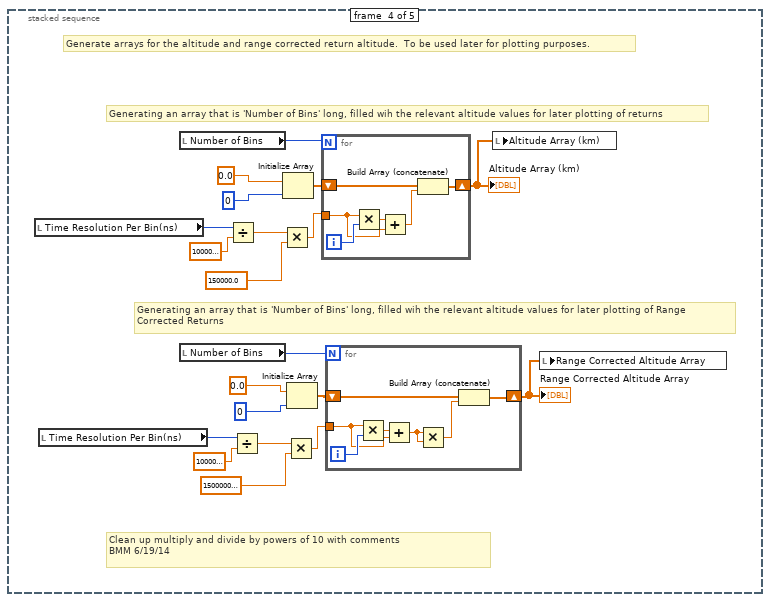
[diagram p12: hidden frame]
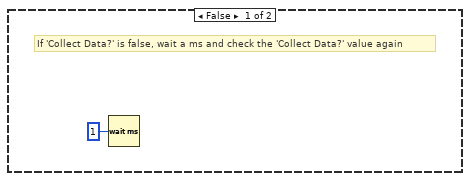
[diagram p13: hidden frame]
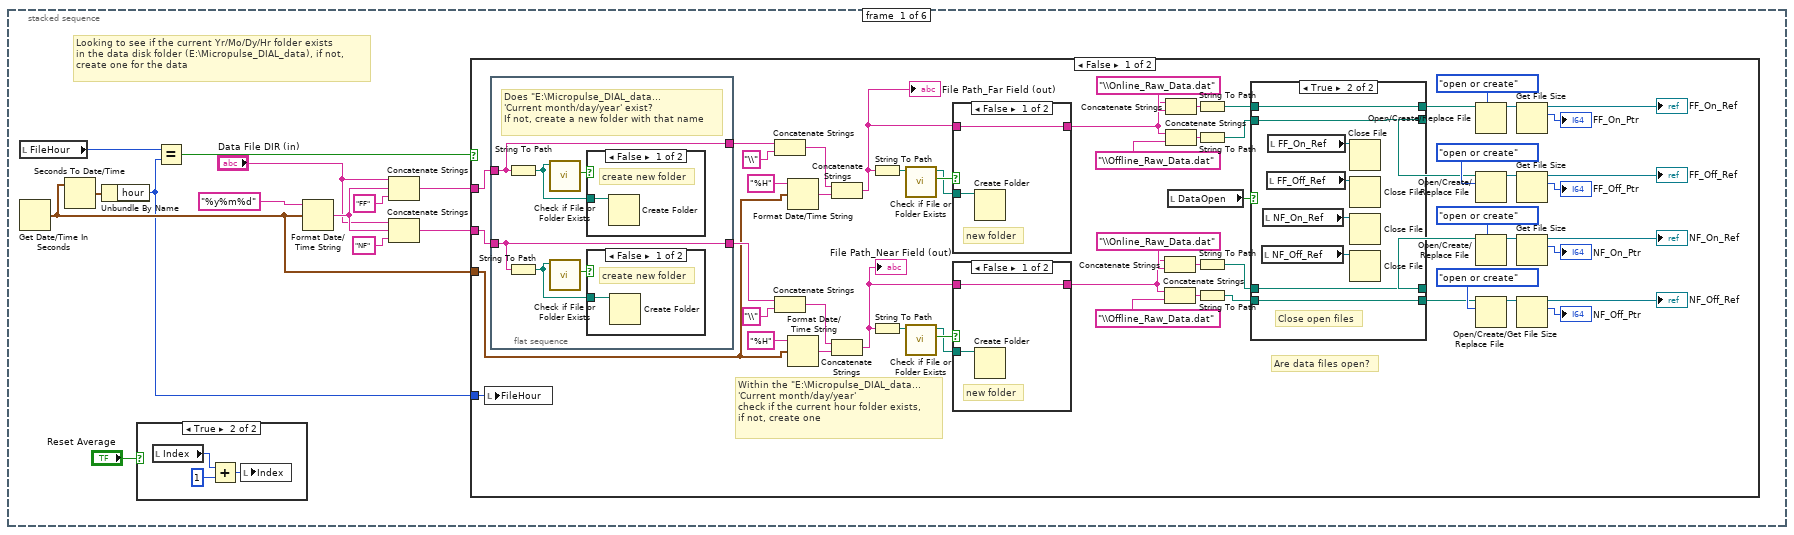
[diagram p14: hidden frame]
diagram:
  # "Frame 0: Initialize the scaler card (and start the MCSC)\nFrame 1: Initialize the DBR's\nFrame 2: (Newport code - REMOVED!!)\nFrame 3: Generate altitude axes for regular and range corrected returns\nFrame 4: Collect data"
  n1 = stacked-sequence {
    tunnel: [_ _ _ _ w98] -> w3
    frame #0 {
      # "Open the Ophir USBI and initialize\nthe functional global power to zero"
      # "Comm Port 5"
      # "Open Bristol WM"
      n2 = disable-structure shown="Enabled" {
        frame Enabled {
          # "Initialization of the AMCS card, this where all of the scaler card parameters\nsuch as number of channels and accumulates is written to the card"
          n3 = stacked-sequence {
            frame #0 {
              # "Sets The Registers Of The Card"
              # "Number Of Channels Used"
              n4 = To Unsigned Long Integer(number="Sync Pulse Polarity") -> (unsigned 32bit integer=w23:u32)
              n5 = To Unsigned Long Integer(number="Pulse A Polarity") -> (unsigned 32bit integer=w27:u32)
              n6 = To Unsigned Long Integer(number="Pulse B Polarity") -> (unsigned 32bit integer=w25:u32)
              n7 = expression code="x*4"(w23) -> (w32:u32)
              n8 = expression code="x*2"(w27) -> (w31:u32)
              n9 = expression code="(x-1)*256"(u32 4 ("Number of Channels Used")) -> (w30:u32)
              n10 = expression code="x/10"("Time Resolution Per Bin(ns)") -> (w34:u32)
              n11 = expression code="x/80"("Pulse A Delay(ns)") -> (w41:u32)
              n12 = expression code="x/80"("Pulse B Delay(ns)") -> (w43:u32)
              n13 = expression code="x/10"("Accumulation Delay(ns)") -> (w42:u32)
              n14 = Compound Arithmetic op=ADD(w32, w31, w25, w30) -> (w29:u32)
              n15 = Build Array(w29, "Number of Bins", "Number of Accumulates", w34, w41, w43, w42) -> ()  [unwired: 1 out]
              n16 = local write "ns scale"("Time Resolution Per Bin(ns)") -> ()
              n17 = local write "y offset"("Accumulation Delay(ns)") -> ()
              n18 = local write "bins"("Number of Bins") -> ()
            }
          }
        }
        frame Disabled {
        }
      }
      n19 = local read "WS_On/Off"() -> (w5:bool)
      n20 = local read "Number of Bins"() -> (w10:u32)
      n21 = case shown="True" w5 {
        frame False {
        }
        frame True {
          n22 = call "ADAM6018_2.1.vi"("ADAM6018_Command"=enum16{"Open_Adam", "Read_Adam", "Close_Adam"}."Open_Adam", "IP Address"="IP Address", "Port"="Port") -> ("ADAM_ID"=→"ID_out":refnum<k5>)  [unwired: 10 in, 2 out]
          n23 = call "T_RH_P.vi"("VISA in"="WS visa", "WS_Commands"=enum16{"OpenWS", "ReadTRHP", "CloseWS"}."OpenWS") -> ("TRHP"=→"TRHP":T12)  [unwired: 11 in, 2 out]
        }
      }
      n24 = dll-call lib="C:/H2O_DIAL/LabVIEW-2012/Bristol WM V2_31b/CLDevIface.dll" fn="CLOpenUSBSerialDevice"("commPort"="Bristol In") -> ("return type"=→"Bristol Out":i32)  [unwired: 4 in, 2 out]
      n25 = call "FunctionalGlobals.vi"("FG_Control"=enum16{"Initialize", "PowerRead", "PowerWrite"}."Initialize") -> ()  [unwired: 14 in, 1 out]
      n26 = Decrement(x=w10) -> (x-1=w9:u32)
      n27 = Subtract(x=w9, y="background length") -> (x-y=→"background start":u32)
      n28 = local read "Ophir PM On/Off"() -> (w4:bool)
      n29 = case shown="True" w4 {
        frame False {
        }
        frame True {
          n30 = call "OpenOphir.vi"("error in (no error)"=errorcluster {"status"=FALSE, "code"=0, "source"=""}) -> ("OphirPM"=→"OphirPM":T7)  [unwired: 13 in, 1 out]
        }
      }
      "Index" <- 0 ("Index")
    }
    frame #1 {
      w44 = FALSE ("Boolean")
      # "Test to see if the lasers are on"
      # "Set the TSOA switch to\namplify the ABSORBING\nwavelength"
      # "Initializing the DBR's.  In this frame the online and offline DBR's are set to the front panel specified initial currents and then the Agiltron switch is toggled to the online channel"
      n31 = local write "WM Switch"(w44) -> ()
      n32 = Build Array(w44) -> (w46:bool[])
      n33 = call-poly <vilib>:"DAQmx Write.vi"("task/channels in"=refnum<k21> "BristolWM", "data"=w46) -> ()  [unwired: 11 in, 3 out]
      n34 = call "TL_Driver.vi"("Device In"=refnum<visa-resource-name> "ThorLabs", "Commands"=T9."Open_TL", "Settings"="Settings") -> ("Device Out"=w58:refnum<visa-resource-name>)  [unwired: 9 in, 3 out]
      n35 = call "TL_Driver.vi"("Device In"=w58, "Commands"=T9."Read_Status", "Settings"="Settings") -> ("Device Out"=w55:refnum<visa-resource-name>, "Readings"=w56:T5)  [unwired: 9 in, 2 out]
      "Readings" <- w56
      n36 = Unbundle By Name(w56) -> ("OnLine LD"=w50:bool, "OffLine LD"=w51:bool)
      n37 = Compound Arithmetic op=AND(TRUE, w50, w51) -> (w49:bool)
      n38 = case shown="False" w49 {
        tunnel: w55 -> [w61 w64]
        tunnel: [w61 w64] -> w53
        frame False {
          n39 = One Button Dialog(message="LASERS NOT ON!", button name ("OK")="CONTINUE") -> ()  [unwired: 1 out]
        }
        frame True {
        }
      }
      n40 = call "TL_Driver.vi"("Device In"=w53, "Commands"=T9."Read_Status", "Settings"="Settings") -> ("Readings"=w45:T5)  [unwired: 9 in, 3 out]
      n41 = local write "Readings"(w45) -> ()
      n42 = local write "Settings"("Settings") -> ()
    }
    frame #2 {
      # "NEWPORT CODE REMOVED!!!!"
    }
    frame #3 {
      # "Clean up multiply and divide by powers of 10 with comments\nBMM 6/19/14"
      # "Generating an array that is 'Number of Bins' long, filled wih the relevant altitude values for later plotting of Range \nCorrected Returns"
      # "Generating an array that is 'Number of Bins' long, filled wih the relevant altitude values for later plotting of returns"
      # "Generate arrays for the altitude and range corrected return altitude.  To be used later for plotting purposes."
      n43 = local read "Time Resolution Per Bin(ns)"() -> (w77:u32)
      n44 = local read "Time Resolution Per Bin(ns)"() -> (w67:u32)
      n45 = local read "Number of Bins"() -> (w80:u32)
      n46 = local read "Number of Bins"() -> (w70:u32)
      n47 = Divide(x=w77, y=1000000000.0) -> (x/y=w75:dbl)
      n48 = Divide(x=w67, y=1000000000.0) -> (x/y=w65:dbl)
      n49 = Multiply(x=w75, y=150000.0) -> (x*y=w78:dbl)
      n50 = Initialize Array(0.0, 0) -> (w83:dbl[])
      n51 = Multiply(x=w65, y=150000000.0) -> (x*y=w68:dbl)
      n52 = Initialize Array(0.0, 0) -> (w73:dbl[])
      n53 = for {
        N: w80 -> [_]
        shift-right: [w96] -> w81
        shift-left: w83 -> [w97]
        tunnel: w78 -> [w93]
        i -> [w95]
        n54 = Multiply(x=w93, y=w95) -> (x*y=w94:dbl)
        n55 = Add(x=w94, y=w93) -> (x+y=w92:dbl)
        n56 = Build Array (concatenate)(w97, w92) -> (w96:dbl[])
      }
      "Altitude Array (km)" <- w81
      n57 = for {
        N: w70 -> [_]
        shift-right: [w90] -> w71
        shift-left: w73 -> [w91]
        tunnel: w68 -> [w86]
        i -> [w89]
        n58 = Multiply(x=w86, y=w89) -> (x*y=w87:dbl)
        n59 = Add(x=w87, y=w86) -> (x+y=w85:dbl)
        n60 = Multiply(x=w85, y=w85) -> (x*y=w88:dbl)
        n61 = Build Array (concatenate)(w91, w88) -> (w90:dbl[])
      }
      "Range Corrected Altitude Array" <- w71
      n62 = local write "Altitude Array (km)"(w81) -> ()
      n63 = local write "Range Corrected Altitude Array"(w71) -> ()
    }
    frame #4 {
      # "Frame 4: Collect data from the scaler card and process and file it"
      n64 = while {
        tunnel: ["stop"] -> w98
        i -> [w99]
        stop <- "stop" stop-if-true
        # "While loop continues data collection cycle"
        n65 = case shown="True" "Collect Data?" {
          frame False {
            # "If 'Collect Data?' is false, wait a ms and check the 'Collect Data?' value again"
            n66 = Wait (ms)(milliseconds to wait=u32 1) -> ()  [unwired: 1 out]
          }
          frame True {
            # "Frame 3: Read the offline wavelength and lock if necessary (code not finished), read output power, read offline data, perform calculations and plot/save offline and NRB data, switch to online\nFrame 4: Calculate the absorption cross section (if wavelength, T, or P changed)\nFrame 5: Calculate Water Vapor Number density and plot"
            # "Frame 0: Create folders and file paths for logging the data, initialize averaging index\nFrame 1: Import current pressure and temperature data from COE weather station\nFrame 2: Read the online wavelength and lock if necessary, read online data and output power\n, plot and save online data, switch to offline DBR"
            # "If 'Collect Data?' is true, collect, process, and log data"
            n67 = stacked-sequence {
              frame #0 {
                # "Looking to see if the current Yr/Mo/Dy/Hr folder exists\nin the data disk folder (E:\\Micropulse_DIAL_data), if not,\ncreate one for the data"
                n68 = local read "FileHour"() -> (w112:i32)
                n69 = Get Date/Time In Seconds() -> (seconds since 1Jan1904=w104:timestamp)
                n70 = Seconds To Date/Time(time stamp (now)=w104) -> (date time rec=w114:T13)  [unwired: 1 in]
                n71 = Unbundle By Name(w114) -> ("hour"=w103:i32)
                n72 = case shown="True" "Reset Average" {
                  frame False {
                    n73 = local write "Index"(0 ("Index")) -> ()
                  }
                  frame True {
                    n74 = local read "Index"() -> (w202:i32)
                    n75 = Add(x=w202, y=1) -> (x+y=w201:i32)
                    n76 = local write "Index"(w201) -> ()
                  }
                }
                n77 = Equal?(x=w112, y=w103) -> (x = y?=w113:bool)
                n78 = Format Date/Time String(time format string (%c)="%y%m%d", seconds (now)=w104) -> (date/time string=w108:string)  [unwired: 1 in]
                n79 = Concatenate Strings("Data File DIR (in)", w108, "FF" ("string")) -> (w110:string)
                n80 = Concatenate Strings("Data File DIR (in)", w108, "NF" ("string")) -> (w105:string)
                n81 = case shown="False" w113 {
                  tunnel: w110 -> [w172 _]
                  tunnel: w105 -> [w171 _]
                  tunnel: w104 -> [w158 _]
                  tunnel: w103 -> [w134 _]
                  frame False {
                    # "Are data files open?"
                    # "Within the \"E:\\Micropulse_DIAL_data...\n'Current month/day/year' \ncheck if the current hour folder exists,\nif not, create one"
                    n82 = local write "FileHour"(w134) -> ()
                    n83 = flat-sequence {
                      tunnel: [w192] -> w159
                      tunnel: w172 -> [w191]
                      tunnel: w171 -> [w192]
                      tunnel: [w191] -> w160
                      frame #0 {
                        # "Does \"E:\\Micropulse_DIAL_data...\n'Current month/day/year' exist?\nIf not, create a new folder with that name"
                        n84 = String To Path(string=w191) -> (path=w196:path)
                        n85 = String To Path(string=w192) -> (path=w194:path)
                        n86 = call <vilib>:"Check if File or Folder Exists.vi"("path"=w196) -> ("file or folder exists?"=w195:bool)  [unwired: 8 in, 2 out]
                        n87 = call <vilib>:"Check if File or Folder Exists.vi"("path"=w194) -> ("file or folder exists?"=w193:bool)  [unwired: 8 in, 2 out]
                        n88 = case shown="False" w195 {
                          tunnel: w196 -> [w198 _]
                          frame False {
                            # "create new folder"
                            n89 = Create Folder(path (use dialog)=w198) -> ()  [unwired: 2 in, 3 out]
                          }
                          frame True {
                            # "Folder exists\ndo nothing"
                          }
                        }
                        n90 = case shown="False" w193 {
                          tunnel: w194 -> [w197 _]
                          frame False {
                            # "create new folder"
                            n91 = Create Folder(path (use dialog)=w197) -> ()  [unwired: 2 in, 3 out]
                          }
                          frame True {
                            # "Folder exists\ndo nothing"
                          }
                        }
                      }
                    }
                    n92 = Concatenate Strings(w160, "\\" ("string")) -> (w167:string)
                    n93 = Concatenate Strings(w159, "\\" ("string")) -> (w162:string)
                    n94 = Format Date/Time String(time format string (%c)="%H", seconds (now)=w158) -> (date/time string=w170:string)  [unwired: 1 in]
                    n95 = Format Date/Time String(time format string (%c)="%H", seconds (now)=w158) -> (date/time string=w165:string)  [unwired: 1 in]
                    n96 = Concatenate Strings(w167, w170) -> (w130:string)
                    "File Path_Far Field (out)" <- w130
                    n97 = Concatenate Strings(w162, w165) -> (w131:string)
                    "File Path_Near Field (out)" <- w131
                    n98 = String To Path(string=w130) -> (path=w168:path)
                    n99 = String To Path(string=w131) -> (path=w163:path)
                    n100 = call <vilib>:"Check if File or Folder Exists.vi"("path"=w168) -> ("file or folder exists?"=w157:bool, "dup path"=w155:path)  [unwired: 8 in, 1 out]
                    n101 = call <vilib>:"Check if File or Folder Exists.vi"("path"=w163) -> ("file or folder exists?"=w156:bool, "dup path"=w154:path)  [unwired: 8 in, 1 out]
                    n102 = case shown="False" w157 {
                      tunnel: w155 -> [w189 _]
                      tunnel: w130 -> [w188 w190]
                      tunnel: [w188 w190] -> w128
                      frame False {
                        # "new folder"
                        n103 = Create Folder(path (use dialog)=w189) -> ()  [unwired: 2 in, 3 out]
                      }
                      frame True {
                        # "Folder exists\ndo nothing"
                      }
                    }
                    n104 = case shown="False" w156 {
                      tunnel: w154 -> [w186 _]
                      tunnel: w131 -> [w185 w187]
                      tunnel: [w185 w187] -> w129
                      frame False {
                        # "new folder"
                        n105 = Create Folder(path (use dialog)=w186) -> ()  [unwired: 2 in, 3 out]
                      }
                      frame True {
                        # "Folder exists\ndo nothing"
                      }
                    }
                    n106 = Concatenate Strings(w129, "\\Online_Raw_Data.dat" ("string")) -> (w148:string)
                    n107 = Concatenate Strings(w129, "\\Offline_Raw_Data.dat" ("string")) -> (w147:string)
                    n108 = Concatenate Strings(w128, "\\Online_Raw_Data.dat" ("string")) -> (w153:string)
                    n109 = Concatenate Strings(w128, "\\Offline_Raw_Data.dat" ("string")) -> (w152:string)
                    n110 = local read "DataOpen"() -> (w145:bool)
                    n111 = String To Path(string=w153) -> (path=w144:path)
                    n112 = String To Path(string=w152) -> (path=w143:path)
                    n113 = String To Path(string=w148) -> (path=w142:path)
                    n114 = String To Path(string=w147) -> (path=w141:path)
                    n115 = case shown="True" w145 {
                      tunnel: w144 -> [w176 w180]
                      tunnel: [w176 w180] -> w138
                      tunnel: w143 -> [w175 w179]
                      tunnel: [w175 w179] -> w137
                      tunnel: w142 -> [w174 w178]
                      tunnel: [w174 w178] -> w136
                      tunnel: [w173 w177] -> w135
                      tunnel: w141 -> [w173 w177]
                      frame False {
                        # "No files open\ndo nothing"
                      }
                      frame True {
                        # "Close open files"
                        n116 = local read "NF_Off_Ref"() -> (w182:refnum<file>)
                        n117 = local read "NF_On_Ref"() -> (w181:refnum<file>)
                        n118 = local read "FF_Off_Ref"() -> (w184:refnum<file>)
                        n119 = local read "FF_On_Ref"() -> (w183:refnum<file>)
                        n120 = Close File(refnum=w183) -> ()  [unwired: 1 in, 2 out]
                        n121 = Close File(refnum=w184) -> ()  [unwired: 1 in, 2 out]
                        n122 = Close File(refnum=w181) -> ()  [unwired: 1 in, 2 out]
                        n123 = Close File(refnum=w182) -> ()  [unwired: 1 in, 2 out]
                      }
                    }
                    n124 = Open/Create/Replace File(file path (use dialog)=w138, operation (0:open)=T10."open or create") -> (refnum out=w124:refnum<file>)  [unwired: 4 in, 2 out]
                    n125 = Open/Create/Replace File(file path (use dialog)=w137, operation (0:open)=T10."open or create") -> (refnum out=w125:refnum<file>)  [unwired: 4 in, 2 out]
                    n126 = Open/Create/Replace File(file path (use dialog)=w136, operation (0:open)=T10."open or create") -> (refnum out=w126:refnum<file>)  [unwired: 4 in, 2 out]
                    n127 = Open/Create/Replace File(file path (use dialog)=w135, operation (0:open)=T10."open or create") -> (refnum out=w127:refnum<file>)  [unwired: 4 in, 2 out]
                    n128 = Get File Size(file=w124) -> (refnum out=→"FF_On_Ref":refnum<file>, size (in bytes)=→"FF_On_Ptr":i64)  [unwired: 1 in, 1 out]
                    n129 = Get File Size(file=w125) -> (refnum out=→"FF_Off_Ref":refnum<file>, size (in bytes)=→"FF_Off_Ptr":i64)  [unwired: 1 in, 1 out]
                    n130 = Get File Size(file=w126) -> (refnum out=→"NF_On_Ref":refnum<file>, size (in bytes)=→"NF_On_Ptr":i64)  [unwired: 1 in, 1 out]
                    n131 = Get File Size(file=w127) -> (refnum out=→"NF_Off_Ref":refnum<file>, size (in bytes)=→"NF_Off_Ptr":i64)  [unwired: 1 in, 1 out]
                  }
                  frame True {
                    # "Don't need to do anything!"
                  }
                }
              }
              frame #1 {
                # "Writing and plotting retrieved\nweather parameters"
                # "Matlab script goes online and retrieves most recent press, temp, and relative humidity data \nfrom the weather station on the roof of Cobleigh"
                # "Importing the current weather conditions from the COE weather station"
                n132 = disable-structure shown="Disabled" {
                  frame Disabled {
                    n133 = script code="%try\n%s=urlread('http://www.coe.montana.edu/ee/weather/mostCurrentCSV.php');\n%amin=textscan(s,'%s %s %s %s %s %s %s %s %s %s %s %s %s');\n%data=amin{1}{2};\n%[test remain]=strtok(data,',');\n%remain=str2num(remain);\n%press=remain(3)./1000;\n%temp=remain(5);\n%RH=remain(7);\n%catch\npress=.850;\ntemp=20;\nRH=40;\n%end"() -> ()  [unwired: 1 in, 4 out]
                  }
                  frame Enabled {
                  }
                }
                n134 = local read "WS_On/Off"() -> (w203:bool)
                n135 = case shown="True" w203 {
                  frame False {
                  }
                  frame True {
                    n136 = disable-structure shown="Disabled" {
                      frame Disabled {
                        n137 = call "ADAM6018.vi"("Remote IP Address 2"="ADAM6018 IP") -> ()  [unwired: 10 in, 1 out]
                      }
                      frame Enabled {
                      }
                    }
                    n138 = local read "WS visa"() -> (w213:refnum<visa-resource-name>)
                    n139 = call "T_RH_P.vi"("VISA in"=w213, "WS_Commands"=enum16{"OpenWS", "ReadTRHP", "CloseWS"}."ReadTRHP") -> ("TRHP"=w208:T12)  [unwired: 11 in, 2 out]
                    n140 = local read "ID_out"() -> (w206:refnum<k5>)
                    n141 = Unbundle By Name(w208) -> ("Temp"=→"Temperature (C)":dbl, "RelH"=→"Relative Humdity (%)":dbl, "Press"=→"Pressure (mb)":dbl)
                    n142 = call "ADAM6018_2.1.vi"("ADAM6018_Command"=enum16{"Open_Adam", "Read_Adam", "Close_Adam"}."Read_Adam", "ID_in"=w206) -> ("Temps"=w207:sgl[])  [unwired: 11 in, 2 out]
                    n143 = local write "TRHP"(w208) -> ()
                    n144 = Index Array(array=w207) -> (element #1=→"T_bench":sgl)  [unwired: 8 in, 7 out]
                  }
                }
              }
              frame #2 {
                # "Frame 3: Read, process, and plot online data\nFrame 4: Switch to the offline DBR seed\nFrame 5: Write the data to the folders from Frame 0 of outter sequence"
                # "Frame 0: Read the online wavelength and adjust to locking tolerance if out of range\nFrame 1: Read the output power from the Newport meter, calculate and plot the output pulse energy\nFrame 2: Wait 'Scalar Wait Time' for buffer to clear other wavelength data"
                # "Online"
                n145 = stacked-sequence {
                  frame #0 {
                    # "Read the online wavelength and continue adjusting the online DBR if outside the wavelength tolerance\nuntil it is within tolerance"
                    n146 = while {
                      i -> [w218]
                      stop <- w216 stop-if-true
                      # "Frame 2: Decrement DBR current if above tolerance\nFrame 3: Increment DBR current if below tolerance"
                      # "Frame 0: Read the current wavelength from the wavemeter\nFrame 1: Calculate the difference between desired and actual wavelength"
                      # "Continue reading and adjusting online DBR current until within locking tolerance"
                      n147 = stacked-sequence {
                        tunnel: w218 -> [w220 _ _ _ _]
                        tunnel: [_ _ w227 _ _] -> w217
                        frame #0 {
                          n148 = Equal To 0?(x=w220) -> (x = 0?=w219:bool)
                          n149 = case shown="True" w219 {
                            frame False {
                            }
                            frame True {
                              w221 = FALSE ("Boolean")
                              # "SWITCH to ABSORBING"
                              n150 = Build Array(w221) -> (w222:bool[])
                              n151 = local write "WM Switch"(w221) -> ()
                              n152 = call-poly <vilib>:"DAQmx Write.vi"("task/channels in"=refnum<k21> "BristolWM", "data"=w222) -> ()  [unwired: 11 in, 3 out]
                            }
                          }
                        }
                        frame #1 {
                          # "Read Bristol WM"
                          n153 = local read "Bristol Out"() -> (w224:i32)
                          n154 = dll-call lib="C:/H2O_DIAL/LabVIEW-2012/Bristol WM V2_31b/CLDevIface.dll" fn="CLGetLambdaReading"("devHandle"=w224) -> ("return type"=→"Lambda On Read (nm)":dbl)  [unwired: 4 in, 2 out]
                        }
                        frame #2 {
                          # "If WL difference is within tolerance, stop looping, and illuminate 'Wavelength Lock Online' indicator"
                          # "Calculating the difference between the actual and desired online wavelength"
                          n155 = local read "Lambda On Read (nm)"() -> (w234:dbl)
                          n156 = local read "Online_Tol"() -> (w231:dbl)
                          n157 = Subtract(x=w234, y="Lambda On Set (nm)") -> (x-y=w226:dbl)
                          "WL Difference" <- w226
                          n158 = Multiply(x=-1.0, y=w231) -> (x*y=w232:dbl)
                          n159 = Greater?(x=w226, y=w232) -> (0:w228:bool)
                          n160 = Less?(x=w226, y=w231) -> (x < y?=w229:bool)
                          n161 = And(x=w228, y=w229) -> (x .and. y?=w227:bool)
                          "Wavelength Lock Online" <- w227
                        }
                        frame #3 {
                          # "If the wavelength difference is greater that 0.0002 nm, decrement the \nDBR current by 0.01 mA"
                          n162 = local read "WL Difference"() -> (w237:dbl)
                          n163 = Greater Or Equal?(x=w237, y="Online_Tol") -> (x >= y?=w235:bool)
                          n164 = case shown="True" w235 {
                            frame False {
                              # "Wavelength difference is not greater than 0.0002 nm, do nothing"
                            }
                            frame True {
                              # "Generating a command string\nto decrement the current"
                              # "WL difference is greater than 0.0002 nm,\ndecrement the DBR current by 0.01 mA"
                              n165 = local read "Settings"() -> (w242:T6)
                              n166 = Unbundle By Name(w242) -> ("OnLineTEC"=w244:dbl)
                              n167 = Subtract(x=w244, y=0.00012) -> (x-y=w245:dbl)
                              n168 = Bundle By Name(cluster=w242, "OnLineTEC"=w245, "Module"=T11."On Line TEC") -> (w240:T6)
                              n169 = call "TL_Driver.vi"("Device In"=refnum<visa-resource-name> "ThorLabs", "Commands"=T9."SET", "Settings"=w240) -> ("Readings"=w238:T5)  [unwired: 9 in, 3 out]
                              n170 = local write "Settings"(w240) -> ()
                              n171 = local write "Readings"(w238) -> ()
                            }
                          }
                        }
                        frame #4 {
                          # "If the wavelength difference is less that 0.0002 nm, increment the \nDBR current by 0.01 mA"
                          n172 = local read "WL Difference"() -> (w251:dbl)
                          n173 = local read "Online_Tol"() -> (w249:dbl)
                          n174 = Multiply(x=-1.0, y=w249) -> (x*y=w247:dbl)
                          n175 = Less Or Equal?(x=w251, y=w247) -> (x <= y?=w250:bool)
                          n176 = case shown="True" w250 {
                            frame False {
                              # "WL difference is no <= to -0.0002 nm, do nothing"
                            }
                            frame True {
                              # "WL difference is < -0.0002,\nincrement the DBR current by 0.01 mA"
                              # "Generating a command string\nto decrement the current"
                              n177 = local read "Settings"() -> (w256:T6)
                              n178 = Unbundle By Name(w256) -> ("OnLineTEC"=w258:dbl)
                              n179 = Add(x=w258, y=0.00012) -> (x+y=w259:dbl)
                              n180 = Bundle By Name(cluster=w256, "OnLineTEC"=w259, "Module"=T11."On Line TEC") -> (w253:T6)
                              n181 = call "TL_Driver.vi"("Device In"=refnum<visa-resource-name> "ThorLabs", "Commands"=T9."SET", "Settings"=w253) -> ("Readings"=w252:T5)  [unwired: 9 in, 3 out]
                              n182 = local write "Settings"(w253) -> ()
                              n183 = local write "Readings"(w252) -> ()
                            }
                          }
                        }
                      }
                      n184 = Or(x=w217, y="Cancel online") -> (x .or. y?=w216:bool)
                    }
                  }
                  frame #1 {
                    # "Reading the output power of the laser transmitter from the Ophir power meter, once read, convert to corresponding pulse energy and plot"
                    n185 = local read "Ophir PM On/Off"() -> (w261:bool)
                    n186 = case shown="True" w261 {
                      frame False {
                      }
                      frame True {
                        # "Plotting the online and offling pulse energies"
                        # "Converting to pulse energy, assumes 5 percent pickoff"
                        n187 = local read "OphirPM"() -> (w266:T7)
                        n188 = call "OphirRead.vi"("OphirPM"=w266) -> ("Power (W)"=w262:dbl, "Ophir Samples"=→"Ophir Samples":i32)  [unwired: 12 in, 1 out]
                        "Average Diode Power" <- w262
                        n189 = Multiply(x=w262, y=1000.0) -> (x*y=w270:dbl)
                        n190 = Divide(x=w270, y="energy scale") -> (x/y=w268:dbl)
                        n191 = Divide(x=w268, y="PRF (kHz)") -> (x/y=w263:dbl)
                        n192 = Bundle(w263) -> (→"Pulse Energy (Micro Joule)":cluster{dbl})  [unwired: 1 in]
                      }
                    }
                  }
                  frame #2 {
                    # "Wait 'Scalar Wait Time' for the next available batch of scalar card data"
                    n193 = local read "AMCS_Profile"() -> (w272:i32)
                    n194 = disable-structure shown="Disabled" {
                      frame Disabled {
                        # "Waiting 'Scalar Wait Time'"
                        n195 = Wait (ms)(milliseconds to wait="Scalar Wait Time (disabled)") -> ()  [unwired: 1 out]
                      }
                      frame Enabled {
                      }
                    }
                    n196 = while {
                      tunnel: [w279] -> w273
                      tunnel: [w275] -> _
                      tunnel: w272 -> [w275]
                      stop <- w277 stop-if-true
                      n197 = global read "AMCS_Data.vi" "AMCS_Profile"() -> (w279:i32)
                      n198 = Wait (ms)(milliseconds to wait=u32 10) -> ()  [unwired: 1 out]
                      n199 = Equal?(x=w279, y=w275) -> (x = y?=w278:bool)
                      n200 = case shown="False" w278 {
                        tunnel: [TRUE FALSE] -> w277
                        frame False {
                        }
                        frame True {
                        }
                      }
                    }
                    "AMCS_Profile" <- w273
                  }
                  frame #3 {
                    # "convert time per range bin to meters\nand calculate smoothed bins using\nsmoothing range"
                    # "Plotting online cross section and smoothed online data"
                    # "Calculate the bin by bin mean of the data"
                    # "Collect 'Integration Period (Seconds)' number\nof scalar data"
                    # "Reading, processing, and plotting the online data"
                    n201 = local read "Data Reads (number of loops)"() -> (w307:i32)
                    n202 = for {
                      N: w307 -> [_]
                      tunnel: [w327] -> w319 mode=indexing
                      tunnel: [w328] -> w299 mode=indexing
                      # "Scalar Data is retrieved from Global \nVariable that scaler.vi is writing to,"
                      n203 = disable-structure shown="Disabled" {
                        frame Disabled {
                          n204 = global read "Scalar_Data.vi" "Scalar Data  3"() -> ()  [unwired: 1 out]
                          n205 = global read "Scalar_Data.vi" "Scalar Data"() -> ()  [unwired: 1 out]
                        }
                        frame Enabled {
                        }
                      }
                      n206 = global read "AMCS_Data.vi" "AMCS_Data"() -> (w331:u16[][])
                      n207 = Index Array(array=w331, index (row) #1=0 ("index (row)"), index (row) #2=2 ("index (row)")) -> (element #1=w327:u16[], element #2=w328:u16[])  [unwired: 2 in]
                    }
                    n208 = Transpose 2D Array(2D array=w319) -> (transposed array=w323:u16[][])
                    n209 = Transpose 2D Array(2D array=w299) -> (transposed array=w305:u16[][])
                    n210 = for {
                      tunnel: w323 -> [w333] mode=indexing
                      tunnel: [w332] -> w324 mode=indexing
                      n211 = call-poly <vilib>:"Mean.vi"("X"=w333) -> ("mean"=w332:dbl)  [unwired: 1 out]
                    }
                    n212 = for {
                      tunnel: w305 -> [w326] mode=indexing
                      tunnel: [w325] -> w306 mode=indexing
                      n213 = call-poly <vilib>:"Mean.vi"("X"=w326) -> ("mean"=w325:dbl)  [unwired: 1 out]
                    }
                    n214 = local read "bins"() -> (w298:u32)
                    n215 = Array Subset(array=w324, index=1 ("dimension size"), length=w298) -> (w311:dbl[])
                    n216 = Array Subset(array=w306, index=1 ("dimension size"), length=w298) -> (w303:dbl[])
                    n217 = local read "background length"() -> (w288:i32)
                    n218 = local read "background start"() -> (w289:u32)
                    n219 = Array Size(array=w311) -> (size(s)=w308:i32)
                    n220 = Array Size(array=w303) -> (size(s)=w300:i32)
                    n221 = Initialize Array(1.0 ("element"), w308) -> (w310:dbl[])
                    n222 = Initialize Array(1.0 ("element"), w300) -> (w302:dbl[])
                    n223 = Multiply(x=w311, y=w310) -> (x*y=w312:dbl[])
                    "On-Line Bin Readings" <- w312
                    n224 = Multiply(x=w303, y=w302) -> (x*y=w292:dbl[])
                    "On-Line Bin Readings 2" <- w292
                    n225 = local read "Total DIAL Integration Time (Minutes)"() -> (w315:i32)
                    n226 = local read "Time Resolution Per Bin(ns)"() -> (w284:u32)
                    n227 = Array Subset(array=w312, index=w289, length=w288) -> (w321:dbl[])
                    n228 = Array Subset(array=w292, index=w289, length=w288) -> (w294:dbl[])
                    n229 = call-poly <vilib>:"Mean.vi"("X"=w321) -> ("mean"=w320:dbl)  [unwired: 1 out]
                    n230 = call-poly <vilib>:"Mean.vi"("X"=w294) -> ("mean"=w295:dbl)  [unwired: 1 out]
                    n231 = Divide(x=w315, y=w307) -> (x/y=w313:dbl)
                    n232 = local read "Index"() -> (w293:i32)
                    n233 = Subtract(x=w312, y=w320) -> (x-y=w317:dbl[])
                    n234 = Subtract(x=w292, y=w295) -> (x-y=w296:dbl[])
                    n235 = To Double Precision Float(number=w284) -> (double precision float=w285:dbl)
                    n236 = Multiply(x=w313, y=60.0) -> (x*y=w290:dbl)
                    n237 = Multiply(x=w285, y=0.15) -> (x*y=w287:dbl)
                    n238 = call "Ring Buffer Online Far.vi"("Index"=w293, "Profiles to Average"=w290, "Input Array"=w317) -> ("AvgArray"=w316:dbl[])  [unwired: 7 in, 1 out]
                    n239 = call "Ring Buffer Online Near.vi"("Index"=w293, "Profiles to Average"=w290, "Input Array"=w296) -> ("AvgArray"=w297:dbl[])  [unwired: 7 in, 1 out]
                    n240 = Divide(x="Smoothing Range", y=w287) -> (x/y=w282:dbl)
                    "Smoothed Bins" <- w282
                    n241 = call "Smooth Arrray.vi"("smooth size"=w282, "Raw Array"=w316) -> ("Smoothed Array"=→"On-Line  Smoothed":dbl[])  [unwired: 9 in]
                    n242 = call "Smooth Arrray.vi"("smooth size"=w282, "Raw Array"=w297) -> ("Smoothed Array"=→"On-Line Smoothed 2":dbl[])  [unwired: 9 in]
                    n243 = disable-structure shown="Disabled" {
                      frame Disabled {
                        n244 = script code="format long;\ncounts=sum(Online);\nif counts >=0.5e6\ntime=time;\nelse\ntime=time\nend"() -> ()  [unwired: 3 in, 2 out]
                      }
                      frame Enabled {
                      }
                    }
                  }
                  frame #4 {
                    # "CODE REMOVED!!"
                    # "Toggling the Agiltron switch to the offline DBR seed laser"
                  }
                  frame #5 {
                    # "Save the recently collected online data if 'Save Data?' is true"
                    n245 = case shown="True" "Save Data?" {
                      frame False {
                        # "'Save Data?' is false, do nothing"
                      }
                      frame True {
                        # "'Save Data?' is true, save onfline data to the Data Disk"
                        # "Write only one copy of data at this time"
                        # "Retrieve Julian Date"
                        n246 = local read "Readings"() -> (w342:T5)
                        n247 = local read "Time Resolution Per Bin(ns)"() -> (w340:u32)
                        n248 = local read "Number of Accumulates"() -> (w338:u32)
                        n249 = local read "Number of Bins"() -> (w339:u32)
                        n250 = local write "DataOpen"(TRUE ("DataOpen")) -> ()
                        n251 = local read "Lambda On Read (nm)"() -> (w364:dbl)
                        n252 = local read "On-Line Bin Readings 2"() -> (w362:dbl[])
                        n253 = local read "On-Line Bin Readings"() -> (w366:dbl[])
                        n254 = local read "Average Diode Power"() -> (w363:dbl)
                        n255 = Unbundle By Name(w342) -> ("OnLineLD"=w341:dbl)
                        n256 = To Double Precision Float(number=w340) -> (double precision float=w337:dbl)
                        n257 = To Double Precision Float(number=w339) -> (double precision float=w336:dbl)
                        n258 = To Double Precision Float(number=w338) -> (double precision float=w335:dbl)
                        n259 = call "Julian_Date_2.vi"() -> ("Julian Date"=w365:dbl)  [unwired: 11 in]
                        n260 = Build Array (concatenate)(w365, w364, w341, w363, w337, w336, w335, w366) -> (w357:dbl[])
                        n261 = Build Array (concatenate)(w365, w364, w341, w363, w337, w336, w335, w362) -> (w347:dbl[])
                        n262 = local read "NF_On_Ref"() -> (w345:refnum<file>)
                        n263 = local read "FF_On_Ref"() -> (w361:refnum<file>)
                        n264 = local read "NF_On_Ptr"() -> (w346:i64)
                        n265 = local read "FF_On_Ptr"() -> (w360:i64)
                        n266 = Set File Position(offset (in bytes) (0)=w360, refnum=w361) -> (refnum out=w358:refnum<file>, error out=w355:errorcluster)  [unwired: 2 in]
                        n267 = Set File Position(offset (in bytes) (0)=w346, refnum=w345) -> (refnum out=w351:refnum<file>, error out=w349:errorcluster)  [unwired: 2 in]
                        n268 = Write to Binary File(file (use dialog)=w351, data=w347, error in=w349, 5:FALSE ("prepend array or string size? (T)")) -> (refnum out=w350:refnum<file>, error out=w348:errorcluster)  [unwired: 2 in, 1 out]
                        n269 = Write to Binary File(file (use dialog)=w358, data=w357, error in=w355, 5:FALSE ("prepend array or string size? (T)")) -> (refnum out=w356:refnum<file>, error out=w354:errorcluster)  [unwired: 2 in, 1 out]
                        n270 = Get File Position(4:w348, 7:w350) -> (2:w344:i64)  [unwired: 2 out]
                        n271 = Get File Position(4:w354, 7:w356) -> (2:w353:i64)  [unwired: 2 out]
                        n272 = local write "NF_On_Ptr"(w344) -> ()
                        n273 = local write "FF_On_Ptr"(w353) -> ()
                      }
                    }
                  }
                }
              }
              frame #3 {
                # "Frame 3: Read offline data, calculate aerosol data, and plot offline and normalized relative backscatter\nFrame 4: Swich to online DBR\nFrame 5: Save the offline data and related information"
                # "Frame 0: Read the offline wavelength and lock if necessary, though code is not finished to do so\nFrame 1: Read the output power from the Newport power meter\nFrame 2: Wait 'Scalar Wait Time' for buffers to clear of online contiminated data"
                # "offline"
                n274 = stacked-sequence {
                  frame #0 {
                    # "Every 60 data collection cycles, read the offline DBR wavelength, and if outside of wavelength tolerance, adjust DBR current until within tolerance"
                    n275 = local read "L_Count"() -> (w368:i32)
                    n276 = Quotient & Remainder(x=w368, y=60.0) -> (x-y*floor(x/y)=w369:dbl)  [unwired: 1 out]
                    n277 = Equal To 0?(x=w369) -> (x = 0?=w367:bool)
                    n278 = case shown="True" w367 {
                      frame False {
                      }
                      frame True {
                        n279 = while {
                          i -> [w374]
                          stop <- w372 stop-if-true
                          # "Frame 5 Increment ofline DBR current if below tolerance\nFrame 6: update ILX settings to front pannel"
                          # "Frame 3: Calculating the wavelength difference\nFrame 4:Decrement offline DBR current if above tolerance"
                          # "Frame 0: Read the offline laser wavelength (settle if t=0)"
                          n280 = stacked-sequence {
                            tunnel: w374 -> [w376 _ _ _ _]
                            tunnel: [_ _ w386 _ _] -> w373
                            frame #0 {
                              n281 = Equal To 0?(x=w376) -> (x = 0?=w375:bool)
                              n282 = case shown="True" w375 {
                                frame False {
                                }
                                frame True {
                                w377 = TRUE ("Boolean")
                                # "SWITCH to NON-ABSORBING and wait to settle"
                                n283 = Build Array(w377) -> (w382:bool[])
                                n284 = local write "WM Switch"(w377) -> ()
                                n285 = call-poly <vilib>:"DAQmx Write.vi"("task/channels in"=refnum<k21> "BristolWM", "data"=w382) -> ()  [unwired: 11 in, 3 out]
                                n286 = call "TL_Driver.vi"("Device In"=refnum<visa-resource-name> "ThorLabs", "Commands"=T9."Read_Status") -> ("Readings"=w380:T5)  [unwired: 10 in, 3 out]
                                n287 = local write "Readings"(w380) -> ()
                                n288 = Wait (ms)(milliseconds to wait=u32 3200) -> ()  [unwired: 1 out]
                                }
                              }
                            }
                            frame #1 {
                              # "Read Bristol WM"
                              n289 = local read "Bristol Out"() -> (w384:i32)
                              n290 = dll-call lib="C:/H2O_DIAL/LabVIEW-2012/Bristol WM V2_31b/CLDevIface.dll" fn="CLGetLambdaReading"("devHandle"=w384) -> ("return type"=→"Lambda Off Read (nm)":dbl)  [unwired: 4 in, 2 out]
                            }
                            frame #2 {
                              # "Once locked, stop looping and illuminate 'Wavelength Lock Offline'"
                              # "While loop continues locking process until the wavelength is within tolerance"
                              # "Calculating the difference between the actual and desired \noffline wavelength"
                              n291 = local read "Lambda Off Read (nm)"() -> (w394:dbl)
                              n292 = Subtract(x=w394, y="Lambda Off Set (nm)") -> (x-y=w387:dbl)
                              "WL Difference off" <- w387
                              n293 = local read "Offline_Tol"() -> (w391:dbl)
                              n294 = Multiply(x=-1.0, y=w391) -> (x*y=w392:dbl)
                              n295 = Greater?(x=w387, y=w392) -> (0:w388:bool)
                              n296 = Less?(x=w387, y=w391) -> (x < y?=w389:bool)
                              n297 = And(x=w388, y=w389) -> (x .and. y?=w386:bool)
                              "Wavelength Lock Offline" <- w386
                              n298 = case shown="True" w386 {
                                frame False {
                                }
                                frame True {
                                w395 = FALSE ("Boolean")
                                # "SWITCH back to ABSORBING and wait to settle"
                                n299 = Build Array(w395) -> (w397:bool[])
                                n300 = local write "WM Switch"(w395) -> ()
                                n301 = call-poly <vilib>:"DAQmx Write.vi"("task/channels in"=refnum<k21> "BristolWM", "data"=w397) -> ()  [unwired: 11 in, 3 out]
                                n302 = Wait (ms)(milliseconds to wait=u32 3200) -> ()  [unwired: 1 out]
                                }
                              }
                            }
                            frame #3 {
                              # "Would adjust the offline wavelength if code was finished"
                              n303 = local read "WL Difference off"() -> (w401:dbl)
                              n304 = Greater Or Equal?(x=w401, y="Offline_Tol") -> (x >= y?=w399:bool)
                              n305 = case shown="True" w399 {
                                frame False {
                                # "WL difference is not out of range, do nothing"
                                }
                                frame True {
                                # "Generating a command string\nto decrement the current"
                                # "WL difference is greater than 0.0002 nm,\ndecrement the DBR current by 0.01 mA"
                                # "WL difference is out of range, this is where you would decrement\nthe laser current"
                                n306 = local read "Settings"() -> (w406:T6)
                                n307 = Unbundle By Name(w406) -> ("OffLineTEC"=w407:dbl)
                                n308 = Subtract(x=w407, y=0.00012) -> (x-y=w408:dbl)
                                n309 = Bundle By Name(cluster=w406, "OffLineTEC"=w408, "Module"=T11."Off Line TEC") -> (w405:T6)
                                n310 = call "TL_Driver.vi"("Device In"=refnum<visa-resource-name> "ThorLabs", "Commands"=T9."SET", "Settings"=w405) -> ("Readings"=w402:T5)  [unwired: 9 in, 3 out]
                                n311 = local write "Settings"(w405) -> ()
                                n312 = local write "Readings"(w402) -> ()
                                }
                              }
                            }
                            frame #4 {
                              # "This is where you would increment the offline current if below tolerance"
                              n313 = local read "Offline_Tol"() -> (w412:dbl)
                              n314 = local read "WL Difference off"() -> (w415:dbl)
                              n315 = Multiply(x=-1.0, y=w412) -> (x*y=w411:dbl)
                              n316 = Less Or Equal?(x=w415, y=w411) -> (x <= y?=w414:bool)
                              n317 = case shown="True" w414 {
                                frame False {
                                # "WL difference is not outisde tolerance, do nothing"
                                }
                                frame True {
                                # "Generating a command string\nto decrement the current"
                                # "WL difference is less than 0.0002 nm,\nincrement the DBR current by 0.01 mA"
                                # "Incrementing the current if below tolerance"
                                n318 = local read "Settings"() -> (w419:T6)
                                n319 = Unbundle By Name(w419) -> ("OffLineTEC"=w421:dbl)
                                n320 = Add(x=w421, y=0.00012) -> (x+y=w422:dbl)
                                n321 = Bundle By Name(cluster=w419, "OffLineTEC"=w422, "Module"=T11."Off Line TEC") -> (w420:T6)
                                n322 = call "TL_Driver.vi"("Device In"=refnum<visa-resource-name> "ThorLabs", "Commands"=T9."SET", "Settings"=w420) -> ("Readings"=w416:T5)  [unwired: 9 in, 3 out]
                                n323 = local write "Settings"(w420) -> ()
                                n324 = local write "Readings"(w416) -> ()
                                }
                              }
                            }
                          }
                          n325 = Or(x=w373, y="Cancel Offline") -> (x .or. y?=w372:bool)
                        }
                      }
                    }
                  }
                  frame #1 {
                    # "CODE REMOVED!!!"
                    # "Reading the output power of the laser transmitter from the Ophir power meter, once read, convert to corresponding pulse energy and plot"
                  }
                  frame #2 {
                    # "Added in the ability to interactively control the ThorLab  setting (just etalon temp for now)"
                    # "CODE REMOVED!!!"
                    # "Wait 'Scalar Wait Time' for buffers to clear of online contiminated offline data"
                    n326 = event shown="[3] \"Settings.OffLineLD\": Value Change" {
                      selector: _ -> [_ _ _ _]
                      dyn-events: _ -> [_ _ _ _]
                      timeout: 1 -> [_ _ _ _]
                      event Timeout {
                        n327 = event-data() -> ()  [unwired: 1 in, 2 out]
                      }
                      event "Settings.EtalonTEC": Value Change {
                        # "Generating a command string\nto update the etalon"
                        n328 = event-data() -> ()  [unwired: 1 in, 5 out]
                        n329 = local read "Settings"() -> (w430:T6)
                        n330 = Unbundle By Name(w430) -> ("EtalonTEC"=w429:dbl)
                        n331 = Bundle By Name(cluster=w430, "EtalonTEC"=w429, "Module"=T11."Etalon TEC") -> (w432:T6)
                        n332 = call "TL_Driver.vi"("Device In"=refnum<visa-resource-name> "ThorLabs", "Commands"=T9."SET", "Settings"=w432) -> ("Readings"=w431:T5)  [unwired: 9 in, 3 out]
                        n333 = local write "Settings"(w432) -> ()
                        n334 = local write "Readings"(w431) -> ()
                      }
                      event "Settings.OnLineLD": Value Change {
                        # "Generating a command string\nto update the Online LD"
                        n335 = event-data() -> ()  [unwired: 1 in, 5 out]
                        n336 = local read "Settings"() -> (w437:T6)
                        n337 = Unbundle By Name(w437) -> ("OnLineLD"=w436:dbl)
                        n338 = Bundle By Name(cluster=w437, "OnLineLD"=w436, "Module"=T11."On Line LD") -> (w439:T6)
                        n339 = call "TL_Driver.vi"("Device In"=refnum<visa-resource-name> "ThorLabs", "Commands"=T9."SET", "Settings"=w439) -> ("Readings"=w438:T5)  [unwired: 9 in, 3 out]
                        n340 = local write "Settings"(w439) -> ()
                        n341 = local write "Readings"(w438) -> ()
                      }
                      event "Settings.OffLineLD": Value Change {
                        # "Generating a command string\nto update the Offline LD"
                        n342 = event-data() -> ()  [unwired: 1 in, 5 out]
                        n343 = local read "Settings"() -> (w444:T6)
                        n344 = Unbundle By Name(w444) -> ("OffLineLD"=w443:dbl)
                        n345 = Bundle By Name(cluster=w444, "OffLineLD"=w443, "Module"=T11."Off Line LD") -> (w446:T6)
                        n346 = call "TL_Driver.vi"("Device In"=refnum<visa-resource-name> "ThorLabs", "Commands"=T9."SET", "Settings"=w446) -> ("Readings"=w445:T5)  [unwired: 9 in, 3 out]
                        n347 = local write "Settings"(w446) -> ()
                        n348 = local write "Readings"(w445) -> ()
                      }
                    }
                  }
                  frame #3 {
                    w480 = 1 ("dimension size")
                    w483 = 1
                    # "Plotting the normalized relative \nbackscatter"
                    # "Calculating the normalized relative backscatter"
                    # "Calculating/Plotting smoothed data,\ncross sections etc."
                    # "Pick off data with\nout header"
                    # "Calculate mean bin by bin mean"
                    # "Reading in 'Integration Period (Seconds)' of data"
                    # "Read the offline data from the scalar card, perform smoothing, calculate normalized relative backscatter, and plot"
                    # "File path in MATLAB script is of old dial is:\nF:\\Micropulse DIAL\\Micropulse DIAL Matlab\\\nFinal Overlap Function.mat')];"
                    # "Collects Data From Card,\nSends It To The Chart,\nAnd Saves A Copy As A\nFile If Option Selected On\nFront Panel"
                    n349 = for {
                      N: "Data Reads (number of loops)" -> [_]
                      tunnel: [w516] -> w513 mode=indexing
                      tunnel: [w515] -> w495 mode=indexing
                      # "Read in latest scalar card data from \n'Scalar Data' global variable that \nscaler.vi is writing to, then wait 1 sec\nfor next batch of data"
                      n350 = global read "AMCS_Data.vi" "AMCS_Data"() -> (w517:u16[][])
                      n351 = disable-structure shown="Disabled" {
                        frame Disabled {
                          n352 = global read "Scalar_Data.vi" "Scalar Data  2"() -> ()  [unwired: 1 out]
                          n353 = global read "Scalar_Data.vi" "Scalar Data  4"() -> ()  [unwired: 1 out]
                        }
                        frame Enabled {
                        }
                      }
                      n354 = Index Array(array=w517, index (row) #1=1 ("index (row)"), index (row) #2=3 ("index (row)")) -> (element #1=w516:u16[], element #2=w515:u16[])  [unwired: 2 in]
                    }
                    n355 = local read "Total DIAL Integration Time (Minutes)"() -> (w504:i32)
                    n356 = Divide(x=w504, y="Data Reads (number of loops)") -> (x/y=w502:dbl)
                    n357 = local read "Total Aerosol Integration Time (Minutes)"() -> (w506:dbl)
                    n358 = Multiply(x=w502, y=60.0) -> (x*y=w488:dbl)
                    n359 = local read "background length"() -> (w452:i32)
                    n360 = local read "background start"() -> (w453:u32)
                    n361 = Transpose 2D Array(2D array=w513) -> (transposed array=w512:u16[][])
                    n362 = Transpose 2D Array(2D array=w495) -> (transposed array=w494:u16[][])
                    n363 = Divide(x=w506, y="Data Reads (number of loops)") -> (x/y=w507:dbl)
                    n364 = for {
                      tunnel: w512 -> [w523] mode=indexing
                      tunnel: [w522] -> w514 mode=indexing
                      tunnel: w494 -> [w521] mode=indexing
                      tunnel: [w520] -> _ mode=indexing
                      tunnel: [w520] -> w491 mode=indexing
                      n365 = call-poly <vilib>:"Mean.vi"("X"=w523) -> ("mean"=w522:dbl)  [unwired: 1 out]
                      n366 = call-poly <vilib>:"Mean.vi"("X"=w521) -> ("mean"=w520:dbl)  [unwired: 1 out]
                    }
                    n367 = local read "bins"() -> (w481:u32)
                    n368 = Multiply(x=w507, y=60.0) -> (x*y=w471:dbl)
                    n369 = Array Subset(array=w491, index=w480, length=w481) -> (w492:dbl[])
                    "Off-Line Bin Readings 2" <- w492
                    n370 = Array Subset(array=w514, index=w480, length=w481) -> (w490:dbl[])
                    "Off-Line  Bin Readings" <- w490
                    n371 = Array Subset(array=w492, index=w453, length=w452) -> (w493:dbl[])
                    n372 = Array Subset(array=w490, index=w453, length=w452) -> (w511:dbl[])
                    n373 = local read "Smoothed Bins"() -> (w449:dbl)
                    n374 = call-poly <vilib>:"Mean.vi"("X"=w493) -> ("mean"=w459:dbl)  [unwired: 1 out]
                    n375 = call-poly <vilib>:"Mean.vi"("X"=w511) -> ("mean"=w460:dbl)  [unwired: 1 out]
                    n376 = local read "Index"() -> (w470:i32)
                    n377 = Subtract(x=w492, y=w459) -> (x-y=w472:dbl[])
                    n378 = Subtract(x=w490, y=w460) -> (x-y=w486:dbl[])
                    n379 = call "Ring Buffer Offline Far.vi"("Index"=w470, "Profiles to Average"=w488, "Input Array"=w486) -> ("AvgArray"=w509:dbl[], "RingBufferOut"=→"RingBuffer offline far":dbl[][])  [unwired: 7 in]
                    n380 = call "Ring Buffer Aerosol Far.vi"("Index"=w470, "Profiles to Average"=w471, "Input Array"=w486) -> ("AvgArray"=w505:dbl[], "RingBufferOut"=→"RingBuffer aerosol far":dbl[][])  [unwired: 7 in]
                    n381 = call "Ring Buffer Offline Near.vi"("Index"=w470, "Profiles to Average"=w488, "Input Array"=w472) -> ("AvgArray"=w489:dbl[], "RingBufferOut"=→"RingBuffer offline near":dbl[][])  [unwired: 7 in]
                    n382 = call "Ring Buffer Aerosol Near.vi"("Index"=w470, "Profiles to Average"=w471, "Input Array"=w472) -> ("AvgArray"=w468:dbl[], "RingBufferOut"=→"RingBuffer aerosol near":dbl[][])  [unwired: 7 in]
                    n383 = Reshape Array(w486, w480, w481) -> (→"raw counts":dbl[][])
                    n384 = Reshape Array(w472, w480, w481) -> (→"raw counts near":dbl[][])
                    n385 = call "Smooth Arrray.vi"("smooth size"=w449, "Raw Array"=w509) -> ("Smoothed Array"=→"Off-Line Smoothed":dbl[])  [unwired: 9 in]
                    n386 = call "Smooth Arrray.vi"("smooth size"=w449, "Raw Array"=w505) -> ("Smoothed Array"=w479:dbl[])  [unwired: 9 in]
                    "Aerosol Smoothed" <- w479
                    n387 = call "Smooth Arrray.vi"("smooth size"=w449, "Raw Array"=w489) -> ("Smoothed Array"=→"Off-Line Smoothed 2":dbl[])  [unwired: 9 in]
                    n388 = call "Smooth Arrray.vi"("smooth size"=w449, "Raw Array"=w468) -> ("Smoothed Array"=w451:dbl[])  [unwired: 9 in]
                    "Aerosol Smoothed 2" <- w451
                    n389 = local read "Number of Accumulates"() -> (w455:u32)
                    n390 = local read "Temperature (C)"() -> (w501:dbl)
                    n391 = local read "Pressure (mb)"() -> (w500:dbl)
                    n392 = script code="%accum_num=10000;     % scaler card setting number of accumulations\nt_bin = 500e-9                 % scaler card setting time per bin\n%t_d = 37.3e-9;                % APD dead time from spec sheet\n\n% conversion from accumulated counts to count rate  (c/s)\nc_convert = 1./t_bin./accum_num;\nCR_far = p_raw_far.*c_convert;\nCR_near = p_raw_near.*c_convert;\nCR_total_far = (p_raw_far+b_far).*c_convert;\nCR_total_near = (p_raw_near+b_near).*c_convert;\nb_CR_far =b_far.*c_convert;\nb_CR_near =b_near.*c_convert;\n\n% create a range array\nsize_p =  size(p_raw_far,2);\nr = (75:75:size_p*75)./1e3; \n    \n%APD correction factor\n D_far = 1./(1-(t_d*CR_total_far));\n D_near = 1./(1-(t_d*CR_total_near));\n\n %Calculating normalize relative backscatter profile\n nrb_far = CR_far.*D_far.*r.^2.*1e-6;\n nrb_near = CR_near.*D_near.*r.^2.*1e-6;"("E"=6.0 ("Real"), "temp"=w501, "press"=w500, "p_raw_far"=w479, "b_far"=w460, "b_near"=w459, "p_raw_near"=w451, "accum_num"=w455, "t_d"="dead time") -> ("nrb_far"=w474:cdb[], "D_far"=w465:dbl[], "nrb_near"=w473:cdb[], "D_near"=w464:dbl[], "b_CR_far"=w457:dbl, "b_CR_near"=w456:dbl)  [unwired: 1 in, 1 out]
                    n393 = local read "bins"() -> (w482:u32)
                    n394 = local read "Altitude Array (km)"() -> (w476:dbl[])
                    n395 = Bundle(w457, w456) -> (→"?":cluster{dbl, dbl})  [unwired: 1 in]
                    n396 = Build Array(w474, w473) -> (w478:cdb[][])
                    n397 = Build Array(w465, w464) -> (w463:dbl[][])
                    n398 = Reshape Array(w473, w483, w482) -> (→"NRB 2":cdb[][])
                    n399 = Reshape Array(w474, w483, w482) -> (→"NRB":cdb[][])
                    n400 = Build Array(w476, w476) -> (w475:dbl[][])
                    n401 = call "Convert to Dynamic Data7"("2D Array"=w463) -> ("Dynamic Data Type"=w462:dynamicdata)  [unwired: 3 in]
                    n402 = call "Convert to Dynamic Data3"("2D Array"=w478) -> ("Dynamic Data Type"=w477:dynamicdata)  [unwired: 3 in]
                    n403 = call "Convert to Dynamic Data4"("2D Array"=w475) -> ("Dynamic Data Type"=w466:dynamicdata)  [unwired: 3 in]
                    n404 = call "Build XY Graph2"("Y Input"=w466, "X Input"=w477) -> ("XY Graph"=→"NRB plot":cluster{"Y":dbl[], "Y":dbl[]}[])  [unwired: 3 in, 6 out]
                    n405 = call "Build XY Graph4"("Y Input"=w466, "X Input"=w462) -> ("XY Graph"=→"Correction":cluster{"Y":dbl[], "Y":dbl[]}[])  [unwired: 3 in, 6 out]
                  }
                  frame #4 {
                    # "CODE REMOVED!!!"
                    # "Toggle Agiltron switch to online DBR"
                  }
                  frame #5 {
                    # "If 'Save Data?' is true, save all relavant offline info"
                    n406 = local read "Save Data?"() -> (w524:bool)
                    n407 = case shown="True" w524 {
                      frame False {
                        # "'Save Data?' is false, do nothing"
                      }
                      frame True {
                        # "Write only one data file at this time"
                        # "Retrive Julian Date"
                        # "'Save Data?' is true, save offline data to the Data Disk"
                        n408 = local read "Readings"() -> (w526:T5)
                        n409 = local read "Off-Line Bin Readings 2"() -> (w545:dbl[])
                        n410 = local read "Lambda Off Read (nm)"() -> (w547:dbl)
                        n411 = local read "Off-Line  Bin Readings"() -> (w552:dbl[])
                        n412 = local read "Relative Humdity (%)"() -> (w551:dbl)
                        n413 = local read "Temperature (C)"() -> (w549:dbl)
                        n414 = Unbundle By Name(w526) -> ("OffLineLD"=w525:dbl)
                        n415 = local read "T_bench"() -> (w548:sgl)
                        n416 = local read "Pressure (mb)"() -> (w550:dbl)
                        n417 = call "Julian_Date_2.vi"() -> ("Julian Date"=w546:dbl)  [unwired: 11 in]
                        n418 = Build Array (concatenate)(w546, w547, w525, w548, w549, w550, w551, w552) -> (w531:dbl[])
                        n419 = Build Array (concatenate)(w546, w547, w525, w548, w549, w550, w551, w545) -> (w528:dbl[])
                        n420 = local read "FF_Off_Ref"() -> (w533:refnum<file>)
                        n421 = local read "NF_Off_Ref"() -> (w530:refnum<file>)
                        n422 = local read "FF_Off_Ptr"() -> (w532:i64)
                        n423 = local read "NF_Off_Ptr"() -> (w529:i64)
                        n424 = Set File Position(offset (in bytes) (0)=w532, refnum=w533) -> (refnum out=w544:refnum<file>, error out=w542:errorcluster)  [unwired: 2 in]
                        n425 = Set File Position(offset (in bytes) (0)=w529, refnum=w530) -> (refnum out=w540:refnum<file>, error out=w538:errorcluster)  [unwired: 2 in]
                        n426 = Write to Binary File(file (use dialog)=w544, data=w531, error in=w542, 5:FALSE ("prepend array or string size? (T)")) -> (refnum out=w543:refnum<file>, error out=w541:errorcluster)  [unwired: 2 in, 1 out]
                        n427 = Write to Binary File(file (use dialog)=w540, data=w528, error in=w538, 5:FALSE ("prepend array or string size? (T)")) -> (refnum out=w539:refnum<file>, error out=w537:errorcluster)  [unwired: 2 in, 1 out]
                        n428 = Get File Position(4:w541, 7:w543) -> (2:w534:i64)  [unwired: 2 out]
                        n429 = Get File Position(4:w537, 7:w539) -> (2:w527:i64)  [unwired: 2 out]
                        n430 = local write "FF_Off_Ptr"(w534) -> ()
                        n431 = local write "NF_Off_Ptr"(w527) -> ()
                      }
                    }
                  }
                }
              }
              frame #4 {
                n432 = First Call?() -> (First Call?: T/F=w555:bool)
                n433 = Or(x="calculate absorption cross sections", y=w555) -> (x .or. y?=w553:bool)
                n434 = case shown="True" w553 {
                  frame False {
                  }
                  frame True {
                    # "calculate absorption cross sections from HITRAN data base"
                    n435 = local read "Off-Line Smoothed"() -> (w556:dbl[])
                    n436 = local read "Lambda On Read (nm)"() -> (w559:dbl)
                    n437 = local read "Lambda Off Set (nm)"() -> (w562:dbl)
                    n438 = local read "Temperature (C)"() -> (w560:dbl)
                    n439 = local read "Pressure (mb)"() -> (w561:dbl)
                    n440 = script code="hitran = dlmread('C:\\H2O_DIAL\\LabVIEW-2012\\Micropulse DIAL Matlab\\815nm_841nm_HITRAN_2008.csv', ',',[1 1 1676 8]);\n%hitran = dlmread('C:\\H2O_DIAL\\LabVIEW-2012\\Micropulse DIAL Matlab\\824nm_841nm_H2O_Spectral_Calc.csv', ',',[1 1 1209 7]);\n\n%Range vector in meters\nrange = ([75:75:size(Online,2)*75]);\n\nif lambda< 828\nlambda=828.195;\nelse\nlambda=lambda;\nend;\n\n%%\n\n%Voigt profile calculation\nWNmin = 1/(828+4)*1e7;  % 832.0 nm converted to wavenumber\nWNmax = 1/(828-4)*1e7;  % 824.0 nm converted to wavenumber\n\n%Find lines from WNmin to WNmax to calculate voigt profile\nline_indices = hitran(1:size(hitran,1),1)>WNmin & hitran(1:size(hitran,1),1)<WNmax;\n\nline = double(hitran(line_indices, 1:size(hitran,2)));\n\n%Calculate temperature and pressure profile\nT0 = 273+25; % surface temperature\nT0 = 273+T0_C;\nT = T0-0.0065.*range; % set to match the sounding\n\n% pressure in atmospheres\nP0  = 0.83; % surface pressure\nP0  = P0_mb/1000*0.986; %pressure in mb converted to atm\nP = P0.*(T0./T).^-5.5;   % set this value to match sounding\n\nT00 = 296;              % HITRAN reference temperature [K]\nP00 = 1;                % HITRAN reference pressure [atm]\nnu0_0 = line(:,1);      % absorption line center wavenumber from HITRAN [cm^-1]\nS0 = line(:,2);         % initial linestrength from HITRAN [cm^-1/(mol*cm^-2)]   \ngammal0 = line(:,4);    % air-broadened halfwidth at T_ref and P_ref from HITRAN [cm^-1/atm]\ngamma_s = line(:,5);    % self-broadened halfwidth at T_ref and P_ref from HITRAN [cm^-1/atm]\nE = line(:,6);          % ground state transition energy from HITRAN [cm^-1]  \nalpha = line(:,7);      % linewidth temperature dependence factor from HITRAN\ndelta = line(:,8);      % pressure shift from HiTRAN [cm^-1 atm^-1]\n\nnu_on = 1/(lambda)*1e7;\nnu_off = 1/(lambda_off)*1e7;\n\nfor i = 1:size(Online,2); % calculate the absorption cross section at each range\n  \n    nu0 = nu0_0+delta.*(P(i)./P00); % unclear if it should be Pi/P00  \n    gammal = gammal0.*(P(i)./P00).*((T00./T(i)).^alpha);    %Calculate Lorentz lineweidth at P(i) and T(i)\n\n    const.m = 18.015E-3./6.022E23; % mass of a single water molecule\n    const.k_B = 1.3806488e-23; % (J/K)\n    const.c = 299792458; % (m/s) (exact)\n \n    gammad = (nu0).*((2.0.*const.k_B.*T(i).*log(2.0))./(const.m.*const.c^2)).^(0.5);  %Calculate HWHM Doppler linewidth at T(i)\n     \n    % term 1 in the Voigt profile\n    y = (gammal./gammad).*((log(2.0)).^(0.5));\n    \n    % term 2 in the Voigt profile\n    x_on = ((nu_on-nu0)./gammad).*(log(2.0)).^(0.5);\n    x_off = ((nu_off-nu0)./gammad).*(log(2.0)).^(0.5);\n    \n    %setting up Voigt convolution\n    t = (-(size(line,1))/2:1:size(line,1)/2-1); %set up the integration spectral step size\n    t = repmat(t',1,length(x_on))';\n    x_on = repmat(x_on,1,length(t));\n    x_off = repmat(x_off,1,length(t));\n    y = repmat(y,1,length(t));\n    f_on = (exp(-t.^2.0))./(y.^2.0+(x_on-t).^2.0);  % combined Voigt term 1 and 2\n    f_off = (exp(-t.^2.0))./(y.^2.0+(x_off-t).^2.0);\n    %Voigt integration over all of the lines at the on and offline locations\n    z_on = trapz(t(1,:),f_on,2);\n    z_off =  trapz(t(1,:),f_off,2);\n    integral_on = z_on;\n    integral_off = z_off;\n    %Calculate linestrength at temperature T\n    S = S0.*((T00./T(i)).^(1.5)).*exp(1.439.*E.*((1./T00)-(1./T(i))));\n \n    %Calculate the Voigt profile\n    K_on = (y(:,1)./pi).*integral_on;\n    K_off = (y(:,1)./pi).*integral_off;\n    \n    %Calculate the Voigt profile absorption cross section [cm^2]\n    sigmav_on = S.*(1./gammad).*(((log(2.0))./pi).^(0.5)).*K_on; %.*far_wing_on;\n    sigmav_off = S.*(1./gammad).*(((log(2.0))./pi).^(0.5)).*K_off; %.*far_wing_off;\n    \n    %Sum contributions from all of the surrounding lines\n    sigma_on_total(i) = sum(sigmav_on);\n    sigma_off_total(i) = sum(sigmav_off);\n    \nend;"("lambda"=w559, "lambda_off"=w562, "P0_mb"=w561, "T0_C"=w560, "Online"=w556) -> ("sigma_on_total"=→"sigma_on_total":dbl[], "sigma_off_total"=→"sigma_off_total":dbl[])  [unwired: 1 in, 1 out]
                  }
                }
              }
              frame #5 {
                w573 = 1
                # "normalization factor\nfrom 300 to 450m"
                # "OPTICAL DEPTH PLOT"
                # "new rainbow color bar display"
                # "Data Processing Far Channel"
                # "new rainbow color bar display"
                # "Calculating the range resolved water vapor number density and plotting"
                n441 = local read "sigma_off_total"() -> (w596:dbl[])
                n442 = local read "sigma_on_total"() -> (w593:dbl[])
                n443 = local read "On-Line  Smoothed"() -> (w571:dbl[])
                n444 = local read "Off-Line Smoothed"() -> (w570:dbl[])
                n445 = local read "Off-Line Smoothed 2"() -> (w594:dbl[])
                n446 = local read "On-Line Smoothed 2"() -> (w595:dbl[])
                n447 = script code="%Time averaging in seconds.  180 Seconds =3 minutes\ntemporal_average = 180;\n\n%Spatial averaging in bins.  2 bins = 150 meters\nspatial_average = 2;\n\n%Creating r and r+deltar vectors..this can also be acsomplished using the\n%diff command\np_oni = Online(:,1:size(Online,2)-1);\n\np_onii = Online(:,2:size(Online,2));\n\np_offi = Offline(:,1:size(Offline,2)-1);\n\np_offii = Offline(:,2:size(Offline,2));\n\nInside = (p_oni.*p_offii)./(p_onii.*p_offi);\n\ndel_cross = 1./(2.*(sigma_on_total(1:size(Online,2)-1)-sigma_off_total(1:size(Offline,2)-1)).*75*100);\n\ndel_cross(isinf(del_cross)) = 0;\n\n%Calculating Number density\nN = del_cross.*log(Inside);\n\n%Spatial smoothing of the profiles\nfilter1 = ones(1,2)./2;\n\nN_1 = N;\n\nN_1_avg = filter2(filter1,N_1);\n\nfilter1 = ones(1,10)./10;\n\nN_2 = N;\n\nN_2_avg = filter2(filter1,N_2);\n\nN_new = zeros(size(N,1),size(N,2));\n \n%Using different averaging windows for different altitudes \nN_avg=[N_1_avg(:,1:40)';N_2_avg(:,41:size(N,2))']';\n\n\nw = N_avg.*1e6.*18.015./6.022e23"("Online"=w595, "Offline"=w594, "sigma_on_total"=w593, "sigma_off_total"=w596) -> ("N_avg"=w597:cdb[], "w"=w606:cdb[])  [unwired: 1 in, 1 out]
                n448 = script code="%Time averaging in seconds.  180 Seconds = 3 minutes\ntemporal_average = 180;\n\n%Spatial averaging in bins.  2 bins = 150 meters\nspatial_average = 2;\n\n%Creating r and r+deltar vectors..this can also be acsomplished using the\n%diff command\np_oni = Online(:,1:size(Online,2)-1);\n\np_onii = Online(:,2:size(Online,2));\n\np_offi = Offline(:,1:size(Offline,2)-1);\n\np_offii = Offline(:,2:size(Offline,2));\n\nInside = (p_oni.*p_offii)./(p_onii.*p_offi);\n\ndel_cross = 1./(2.*(sigma_on_total(1:size(Online,2)-1)-sigma_off_total(1:size(Offline,2)-1)).*75*100);\n\ndel_cross(isinf(del_cross)) = 0;\n\n%Calculating Number density\nN = del_cross.*log(Inside);\n\n%Spatial smoothing of the profiles\nfilter1 = ones(1,2)./2;\n\nN_1 = N;\n\nN_1_avg = filter2(filter1,N_1);\n\nfilter1 = ones(1,10)./10;\n\nN_2 = N;\n\nN_2_avg = filter2(filter1,N_2);\n\nN_new = zeros(size(N,1),size(N,2));\n \n%Using different averaging windows for different altitudes \nN_avg=[N_1_avg(:,1:40)';N_2_avg(:,41:size(N,2))']';\n\n \nw = N_avg.*1e6.*18.015./6.022e23"("Online"=w571, "Offline"=w570, "sigma_on_total"=w593, "sigma_off_total"=w596) -> ("N_avg"=w602:cdb[], "w"=w603:cdb[])  [unwired: 1 in, 1 out]
                n449 = local read "Time Resolution Per Bin(ns)"() -> (w572:u32)
                n450 = local read "bins"() -> (w598:u32)
                n451 = local read "Altitude Array (km)"() -> (w568:dbl[])
                n452 = Build Array(w603, w606) -> (w609:cdb[][])
                n453 = To Double Precision Float(number=w572) -> (double precision float=w591:dbl)
                n454 = Reshape Array(w602, w573, w598) -> (w613:cdb[][])
                n455 = Reshape Array(w597, w573, w598) -> (w600:cdb[][])
                n456 = Multiply(x=0.15, y=w591) -> (x*y=w589:dbl)
                n457 = Build Array(w602, w597) -> (w607:cdb[][])
                n458 = Divide(x=300.0, y=w589) -> (x/y=w586:dbl)
                n459 = Divide(x=450.0, y=w589) -> (x/y=w585:dbl)
                n460 = Build Array(w568, w568) -> (w592:dbl[][])
                n461 = call "Convert to Dynamic Data5"("2D Array"=w609) -> ("Dynamic Data Type"=w608:dynamicdata)  [unwired: 3 in]
                n462 = call "Convert to Dynamic Data2"("2D Array"=w607) -> ("Dynamic Data Type"=w604:dynamicdata)  [unwired: 3 in]
                n463 = Divide(x=w613, y=1e+17) -> (x/y=→"Water Vapor Number Density":cdb[][])
                n464 = Divide(x=w600, y=1e+17) -> (x/y=→"Water Vapor Number Density 2":cdb[][])
                n465 = call "Convert to Dynamic Data6"("Array"=w568) -> ("Dynamic Data Type"=w569:dynamicdata)  [unwired: 3 in]
                n466 = To Long Integer(number=w586) -> (32bit integer=w584:i32)
                n467 = To Long Integer(number=w585) -> (32bit integer=w583:i32)
                n468 = call "Convert to Dynamic Data"("2D Array"=w592) -> ("Dynamic Data Type"=w605:dynamicdata)  [unwired: 3 in]
                n469 = call "Convert to Dynamic Data8"("2D Array"=w592) -> ("Dynamic Data Type"=w610:dynamicdata)  [unwired: 3 in]
                n470 = Decrement(x=w584) -> (x-1=w581:i32)
                n471 = Decrement(x=w583) -> (x-1=w582:i32)
                n472 = call "Build XY Graph"("Y Input"=w605, "X Input"=w604) -> ("XY Graph"=→"Water Vapor Number Density  2":cluster{"Y":dbl[], "Y":dbl[]}[])  [unwired: 3 in, 6 out]
                n473 = call "Build XY Graph3"("Y Input"=w610, "X Input"=w608) -> ("XY Graph"=→"Absolute Humidity":cluster{"Y":dbl[], "Y":dbl[]}[])  [unwired: 3 in, 6 out]
                n474 = Array Subset(array=w571, index=w581, length=w582) -> (w580:dbl[])
                n475 = Array Subset(array=w570, index=w581, length=w582) -> (w579:dbl[])
                n476 = call-poly <vilib>:"Mean.vi"("X"=w580) -> ("mean"=w578:dbl)  [unwired: 1 out]
                n477 = call-poly <vilib>:"Mean.vi"("X"=w579) -> ("mean"=w577:dbl)  [unwired: 1 out]
                n478 = Divide(x=w578, y=w577) -> (x/y=w576:dbl)
                n479 = Multiply(x=w570, y=w576) -> (x*y=w575:dbl[])
                n480 = Divide(x=w571, y=w575) -> (x/y=w574:dbl[])
                n481 = Natural Logarithm(1:w574) -> (0:w565:dbl[])
                n482 = Multiply(x=-1.0, y=w565) -> (x*y=w564:dbl[])
                n483 = call "Convert to Dynamic Data9"("Array"=w564) -> ("Dynamic Data Type"=w567:dynamicdata)  [unwired: 3 in]
                n484 = call "Build OD Plot"("Y Input"=w569, "X Input"=w567) -> ("XY Graph"=→"Optical Depth":cluster{"Y":dbl[], "Y":dbl[]}[])  [unwired: 3 in, 6 out]
              }
            }
          }
        }
        "L_Count" <- w99
      }
    }
  }
  n485 = case shown="True" w3 {
    frame False {
    }
    frame True {
      # "close data files"
      # "Close Bristol WM"
      n486 = local read "Ophir PM On/Off"() -> (w617:bool)
      n487 = local read "Bristol Out"() -> (w622:i32)
      n488 = local read "NF_Off_Ref"() -> (w618:refnum<file>)
      n489 = local read "NF_On_Ref"() -> (w619:refnum<file>)
      n490 = local read "FF_Off_Ref"() -> (w620:refnum<file>)
      n491 = local read "WS_On/Off"() -> (w616:bool)
      n492 = local read "FF_On_Ref"() -> (w621:refnum<file>)
      n493 = case shown="True" w616 {
        frame False {
        }
        frame True {
          n494 = local read "WS visa"() -> (w627:refnum<visa-resource-name>)
          n495 = local read "ID_out"() -> (w624:refnum<k5>)
          n496 = call "T_RH_P.vi"("VISA in"=w627, "WS_Commands"=enum16{"OpenWS", "ReadTRHP", "CloseWS"}."CloseWS") -> ()  [unwired: 11 in, 3 out]
          n497 = call "ADAM6018_2.1.vi"("ADAM6018_Command"=enum16{"Open_Adam", "Read_Adam", "Close_Adam"}."Close_Adam", "ID_in"=w624) -> ()  [unwired: 11 in, 3 out]
        }
      }
      n498 = case shown="True" w617 {
        frame False {
        }
        frame True {
          n499 = local read "OphirPM"() -> (w623:T7)
          n500 = call "OphirClose.vi"("OphirPM"=w623) -> ()  [unwired: 18 in, 1 out]
        }
      }
      n501 = dll-call lib="C:/H2O_DIAL/LabVIEW-2012/Bristol WM V2_31b/CLDevIFace.dll" fn="CLCloseDevice"("CommPort"=w622) -> ()  [unwired: 5 in, 2 out]
      n502 = Close File(refnum=w621) -> ()  [unwired: 1 in, 2 out]
      n503 = Close File(refnum=w620) -> ()  [unwired: 1 in, 2 out]
      n504 = Close File(refnum=w619) -> ()  [unwired: 1 in, 2 out]
      n505 = Close File(refnum=w618) -> ()  [unwired: 1 in, 2 out]
    }
  }
  "FileHour" <- -1 ("FileHour")
  "DataOpen" <- FALSE
